vi "cDAQ.vi"(9 "Tipo motore":refnum<vi>, 10 "simulazione?":bool=TRUE, 11 "Dati Targa per calcoli":refnum<vi>) -> (0 "error out":errorcluster)   [LabVIEW 2019]
uses:
  <resource>/objmgr/daqmx.rc
  SET SINGLE DO.ctl
  SET SINGLE AO.ctl
  DO List.ctl
  AO List.ctl
  <vilib>/Analysis/NI_AALBase.lvlib
  <vilib>/Analysis/baseanly.llb/Mean (DBL).vi
  SET ARRAY DO.ctl
  SubVI/Global RPM simulati.vi
  SubVI/Global Coppia letta.vi
  <vilib>/DAQmx/read.llb/DAQmx Read (Counter DBL 1Chan 1Samp).vi
  <vilib>/DAQmx/create/channels.llb/DAQmx Create Channel (CI-Position-Angular Encoder).vi
  <vilib>/DAQmx/configure/timing.llb/DAQmx Timing (Implicit).vi
  <vilib>/DAQmx/create/channels.llb/DAQmx Create Channel (CI-Frequency).vi
  <vilib>/DAQmx/configure/timing.llb/DAQmx Timing (Sample Clock).vi
  <vilib>/DAQmx/create/channels.llb/DAQmx Create Channel (AO-Voltage-Basic).vi
  <vilib>/DAQmx/create/channels.llb/DAQmx Create Channel (AI-Voltage-Basic).vi
  <vilib>/DAQmx/create/channels.llb/DAQmx Create Channel (DO-Digital Output).vi
  <vilib>/DAQmx/create/channels.llb/DAQmx Create Channel (AI-Temperature-Thermocouple).vi
  <vilib>/DAQmx/create/channels.llb/DAQmx Create Channel (DI-Digital Input).vi
  <vilib>/DAQmx/write.llb/DAQmx Write (Analog 1D DBL NChan 1Samp).vi
  <vilib>/DAQmx/read.llb/DAQmx Read (Analog 1D DBL NChan 1Samp).vi
  <vilib>/DAQmx/read.llb/DAQmx Read (Digital 1D Bool 1Chan 1Samp).vi
  <vilib>/DAQmx/read.llb/DAQmx Read (Analog 1D Wfm NChan NSamp).vi
  SubVI/EXIT.vi
  <vilib>/DAQmx/write.llb/DAQmx Write (Digital 1D Bool 1Chan 1Samp).vi
  SubVI/angle global.vi
  SET ARRAY AO.ctl
  controls/statoDO_Cdaq.ctl
panel:
  out "Waveform Chart 2":dbl(graph)
  out "x-y":u32
  out "t ciclo effettivo AO":u32
  out "error out 3":errorcluster
  out "Cnom 2":dbl
  out "Waveform Chart 3":dbl(graph)
  out "error CTR 2":errorcluster
  out "error Angle 2":errorcluster
  out "error out 2":errorcluster
  out "t ciclo effettivo ai":u32
  in  "Time filtro(s)":dbl=0.8 format="%#_13g"
  in  "Tab Control":T1(tab)
  in  "counter 4":tag="C2017003Mod7/ctr1"
  in  "counter 3":tag="C2017003Mod7/ctr3"
  in  "stop":bool
  in  "lines 32DI":tag="C2017003Mod1/port0/line0:31"
  in  "physical channels 4TC":tag="C2017003Mod5/ai0:3, C2017003Mod6/ai0:3"
  in  "lines 32DO":tag="C2017003Mod2/port0/line0:31"
  in  "physical channels 4AO":tag="C2017003Mod4/ao0:3"
  in  "physical channels":tag="C2017003Mod3/ai0:3"
  in  "counter 2":tag="C2017003Mod7/ctr0"
  in  "counter":tag="C2017003Mod7/ctr2"
  in  "SET DO":bool
  in  "Cluster SET AO":T2
  in  "SET AO":bool
  in  "Array DO":T5
  out "statoAO":T8
  out "AI":T9
  out "Termocoppie":T10
  out "angle1":bool
  out "freq":dbl format="%0.2f"
  out "rpm":dbl
  out "t ciclo effettivo LF 1 cntr":u32
  out "statoDO":T11
  out "# pending insert":i32
  out "Numeric":i32
  out "# pending insert 2":i32
  out "angle2":bool
  out "freq 2":dbl format="%0.2f"
  out "rpm 2":dbl
  out "t ciclo effettivo LF 1 cntr 2":u32
  out "error DI":errorcluster
  out "error TC":errorcluster
  out "error DO":errorcluster
  out "error AO":errorcluster
  out "error AI":errorcluster
  out "error Angle":errorcluster
  out "error CTR":errorcluster
  out "XY Graph":cluster{"X":dbl, "Y":dbl}[](graph)
  out "Waveform Chart":waveform(dbl)(graph)
  in  "Boolean":bool
  out "Cnom":dbl
  out "String":string
  in  "EXIT":bool
  in  "STOP GENERALE 2":bool
  # "STATO INGRESSI"
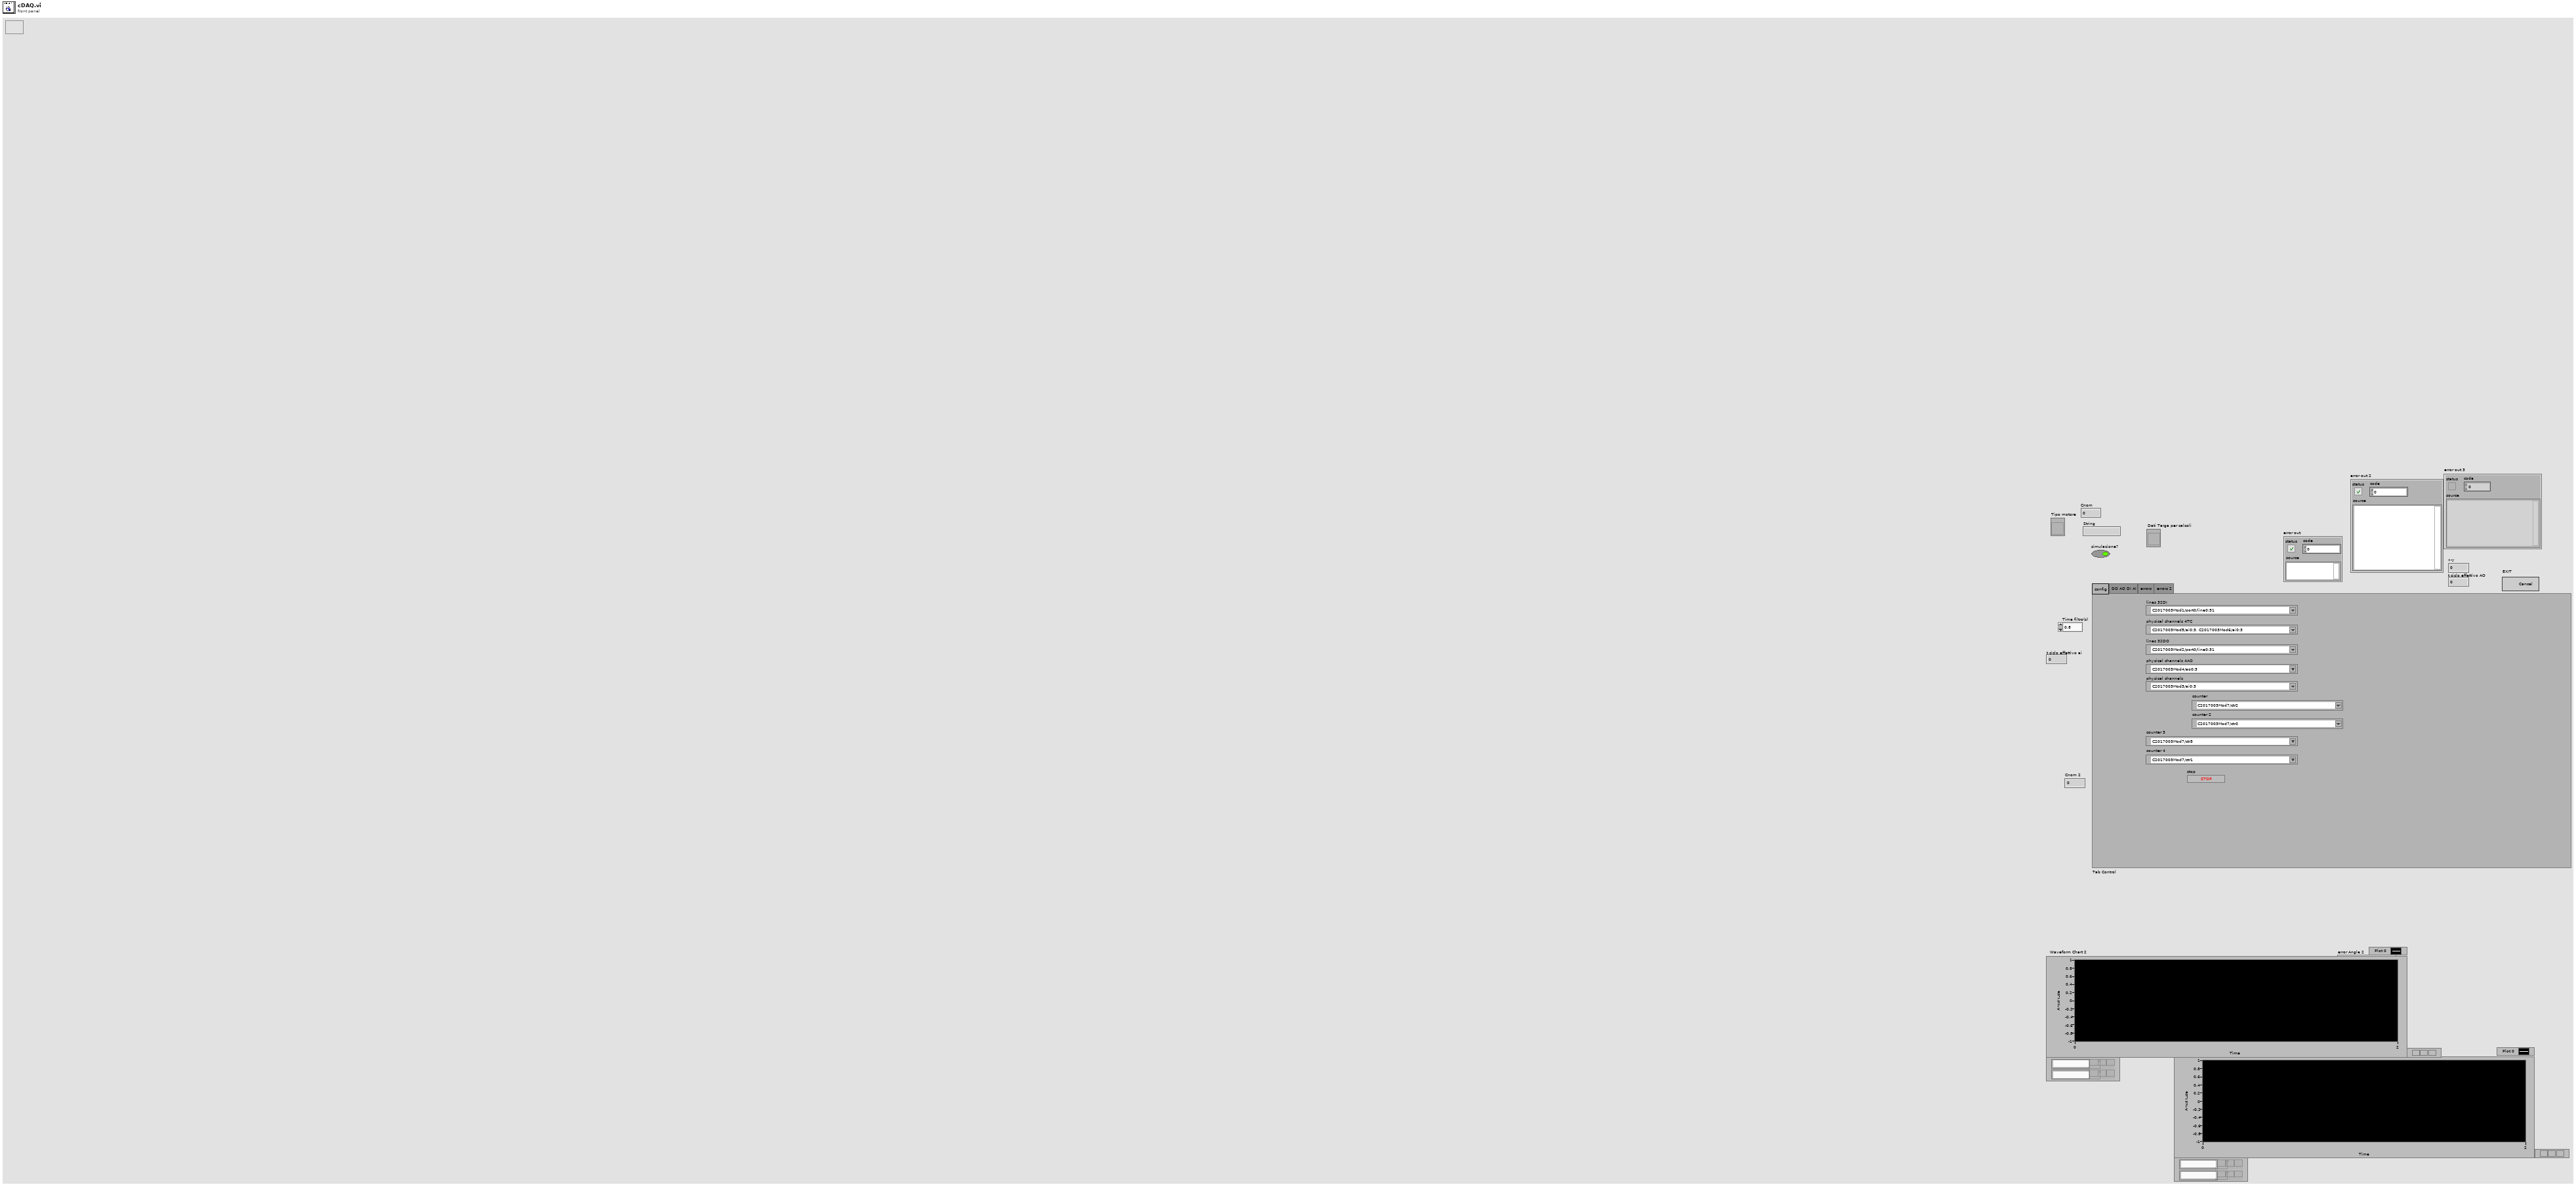
[diagram p1: front panel]
types:
  T1 = enum32{"config", "DO AO DI AI", "errors", "errors 2"}
  T2 = typedef "SET ARRAY AO.ctl" = T3[]
  T3 = typedef "SET SINGLE AO.ctl" = cluster{"AO":T4, "Value":dbl}
  T4 = typedef "AO List.ctl" = enum16{"OFF: ALL AO", "RIF VEL FRENO 1", "RIF VEL FRENO 2", "RIF VEL FRENO 3", "RIF COPPIA FRENO 1", "RIF COPPIA FRENO 2", "RIF COPPIA FRENO 3", "RIF V ALIM 1", "RIF F ALIM 1", "RIF V ALIM 2", "RIF F ALIM 2", "RIF V ALIM 3", "RIF F ALIM 3", "RIF V ALIM 4", "RIF F ALIM 4", "FORZA AO PLC 3", "FORZA AO PLC 2", "FORZA AO PLC 1", "FORZA AO cDAQ", "Configura alimentatore keb", "Tempo rampa keb", "Condensatori", "Exit"}
  T5 = typedef "SET ARRAY DO.ctl" = T6[]
  T6 = typedef "SET SINGLE DO.ctl" = cluster{"DO":T7, "Value":bool}
  T7 = typedef "DO List.ctl" = enum16{"OFF: ALL DO", "*ABILITA freno 1", "*ABILITA freno 2", "*ABILITA freno 3", "*START freno 1", "*START freno 2", "*START freno 3", "*STOP freno 1", "*STOP freno 3", "*STOP freno 2", "*Senso rot freno 1", "*Senso rot freno 2", "*Senso rot freno 3", "*Ctrl velocità freno 1", "*Ctrl velocità freno 2", "*Ctrl velocità freno 3", "*Ctrl coppia freno 1", "*Ctrl coppia freno 2", "*Ctrl coppia freno 3", "*ABILITA alimentatore 1", "*ABILITA alimentatore 2", "*ABILITA alimentatore 3", "*ABILITA alimentatore 4", "*START alimentatore 1", "*START alimentatore 2", "*START alimentatore 3", "*START alimentatore 4", "*STOP alimentatore 1", "*STOP alimentatore 2", "*STOP alimentatore 3", "*STOP alimentatore 4", "SENSO ROT alimentatore 1", "SENSO ROT alimentatore 2", "Abilita LEM 1000A", "Abilita LEM 300A", "Abilita sensori EXT WT", "B1 Seleziona linea 1", "B1 Seleziona linea 2", "B1 Seleziona linea 3", "B1 Seleziona linea 4", "B1 Seleziona linea 5", "B2 Seleziona linea 1", "B2 Seleziona linea 2", "B2 Seleziona linea 3", "B2 Seleziona linea 4", "B2 Seleziona linea 5", "*Reset allarmi", "*Start potenza AC", "*Stop potenza AC", "*Start potenza DC", "*Stop potenza DC", "*Start potenza DC eccit", "*Stop pontenza DC eccit", "Bypass res meter", "2nd canale res meter", "Enable res meter", "*Abilit teler ramo WT", "*Abil teler ramo princ Resit", "*Abil teler ramo 1 Resist", "*Abil teler ramo 2 Resist", "*Abil teler ramo 3 Resist", "*Abil cortocirc avvolgim", "*Controllo torsiometro B1", "*Controllo Torsiom B2", "*Scala torsiometro B1", "*Scala torsiometro B2", "*Collaudo in corso", "*Allarme presente", "Abilitazione elettroserratura", "Exit", "*Abilita collaudo", "*Abilita potenza trifase", "*Abilita potenza monofase", "*Abilita potenza DC", "*Abilita potenza DC eccit", "*Disabilita teleruttori potenza", "Set teleruttori prova a freddo", "Prova a freddo monofase", "Watchdog", "Forza DO PLC 3", "Forza DO PLC 2", "Forza DO PLC 1", "Forza DO cDAQ", "Scala 2000(T) 200(F) res meter", "Seleziona banco 1", "Seleziona banco 2", "Comando azionam in blocco", "Comando azionam reset", "Sensibilità freno 16 32 nm", "Reset Allarmi", "Carico res - Ramo 1", "Carico res - Ramo 2", "Carico res - Ramo 3", "Carico res - Ramo 4", "Carico res - Ramo 5", "Carico res - Ramo 6", "Carico res - Ramo 7", "Carico res - Ramo 8", "Carico res - Ramo 9", "Carico res - Ramo 10", "Carico res - Ramo 11", "Carico res - Start ventilatore", "Carico res - Stop ventilatore", "Abilita potenza solo freno", "Abilita AFE + freno trasc", "Abilita potenza carico resistivo", "Chiudi potenza AFE", "Apri potenza AFE", "Start AFE", "Config Banco2 TDE", "Misura diretto WT", "Ripristina centralina protezioni", "Abilita Scrittura Dati Keb"}
  T8 = cluster{"V eccitaz":dbl, "I eccitaz":dbl, "Rif vel freno":dbl, "Rif coppia freno":dbl}
  T9 = cluster{"Torsiometro":dbl, "V eccitazione":dbl, "I eccitazione":dbl, "Scorta":dbl}
  T10 = cluster{"TC 1":dbl, "TC 2":dbl, "TC 3":dbl, "Tamb (°C)":dbl, "TC 4":dbl, "TC 5":dbl, "TC 6":dbl, "Tamb (°C) 2":dbl}
  T11 = typedef "statoDO_Cdaq.ctl" = cluster{"Scorta 0":bool, "Scorta 1":bool, "Scorta 2":bool, "Scorta 3":bool, "Scorta 4":bool, "Scorta 5":bool, "Scorta 6":bool, "Scorta 7":bool, "Scorta 8":bool, "Scorta 9":bool, "Scorta 10":bool, "Scorta 11":bool, "Scorta 12":bool, "Scorta 13":bool, "Scorta 14":bool, "Scorta 15":bool, "Scorta 16":bool, "Scorta 17":bool, "Scorta 18":bool, "Scorta 19":bool, "Scorta 20":bool, "Scorta 21":bool, "Scorta 22":bool, "Scorta 23":bool, "Scorta 24":bool, "Scorta 25":bool, "Scorta 26":bool, "Scorta 27":bool, "Scorta 28":bool, "Scorta 29":bool, "Scorta 30":bool, "Scorta 31":bool}
  T12 = typedef "Dati targa per calcoli.ctl" = cluster{"trifase":cluster{"I nom (A)":dbl, "C nom (Nm)":dbl, "Npoli":dbl, "V nom (V)":dbl, "RPM nom":dbl}, "Monofase":cluster{"I nom (A)":dbl, "C nom (Nm)":dbl, "Npoli":dbl, "V nom (V)":dbl, "RPM nom":dbl}, "Dc":cluster{"I nom (A)":dbl, "C nom (Nm)":dbl, "V nom (V)":dbl, "RPM nom":dbl}}
  T13 = cluster{"[0]":dbl, "[1]":dbl, "[2]":dbl, "[3]":dbl}
  T14 = cluster{"Motore monofase abil":bool, "Motore trifase abil":bool, "Uscita generale abil":bool, "2nd ch res meter abil":bool, "TA selezionati":bool, "Pulsante Start prova":bool, "Pulsante Stop prova":bool, "Pulsante Reset allarmi":bool, "Secondari TA aperti":bool, "Res meter abil":bool, "Scorta 1":bool, "Scorta 2":bool, "Scorta 3":bool, "Scorta 4":bool, "Scorta 5":bool, "Scorta 6":bool, "Scorta 7":bool, "Scorta 8":bool, "Scorta 9":bool, "Scorta 10":bool, "Scorta 11":bool, "Scorta 12":bool, "Scorta 13":bool, "Scorta 14":bool, "Scorta 15":bool, "Scorta 16":bool, "Scorta 17":bool, "Scorta 18":bool, "Scorta 19":bool, "Scorta 20":bool, "Scorta 21":bool, "Scorta 22":bool}
  T15 = cluster{"data[0]":dbl, "data[1]":dbl, "data[2]":dbl, "data[3]":dbl, "data[4]":dbl, "data[5]":dbl, "data[6]":dbl, "data[7]":dbl}
  T16 = cluster{"[0]":bool, "[1]":bool, "[2]":bool, "[3]":bool, "[4]":bool, "[5]":bool, "[6]":bool, "[7]":bool, "[8]":bool, "[9]":bool, "[10]":bool, "[11]":bool, "[12]":bool, "[13]":bool, "[14]":bool, "[15]":bool, "[16]":bool, "[17]":bool, "[18]":bool, "[19]":bool, "[20]":bool, "[21]":bool, "[22]":bool, "[23]":bool, "[24]":bool, "[25]":bool, "[26]":bool, "[27]":bool, "[28]":bool, "[29]":bool, "[30]":bool, "[31]":bool}
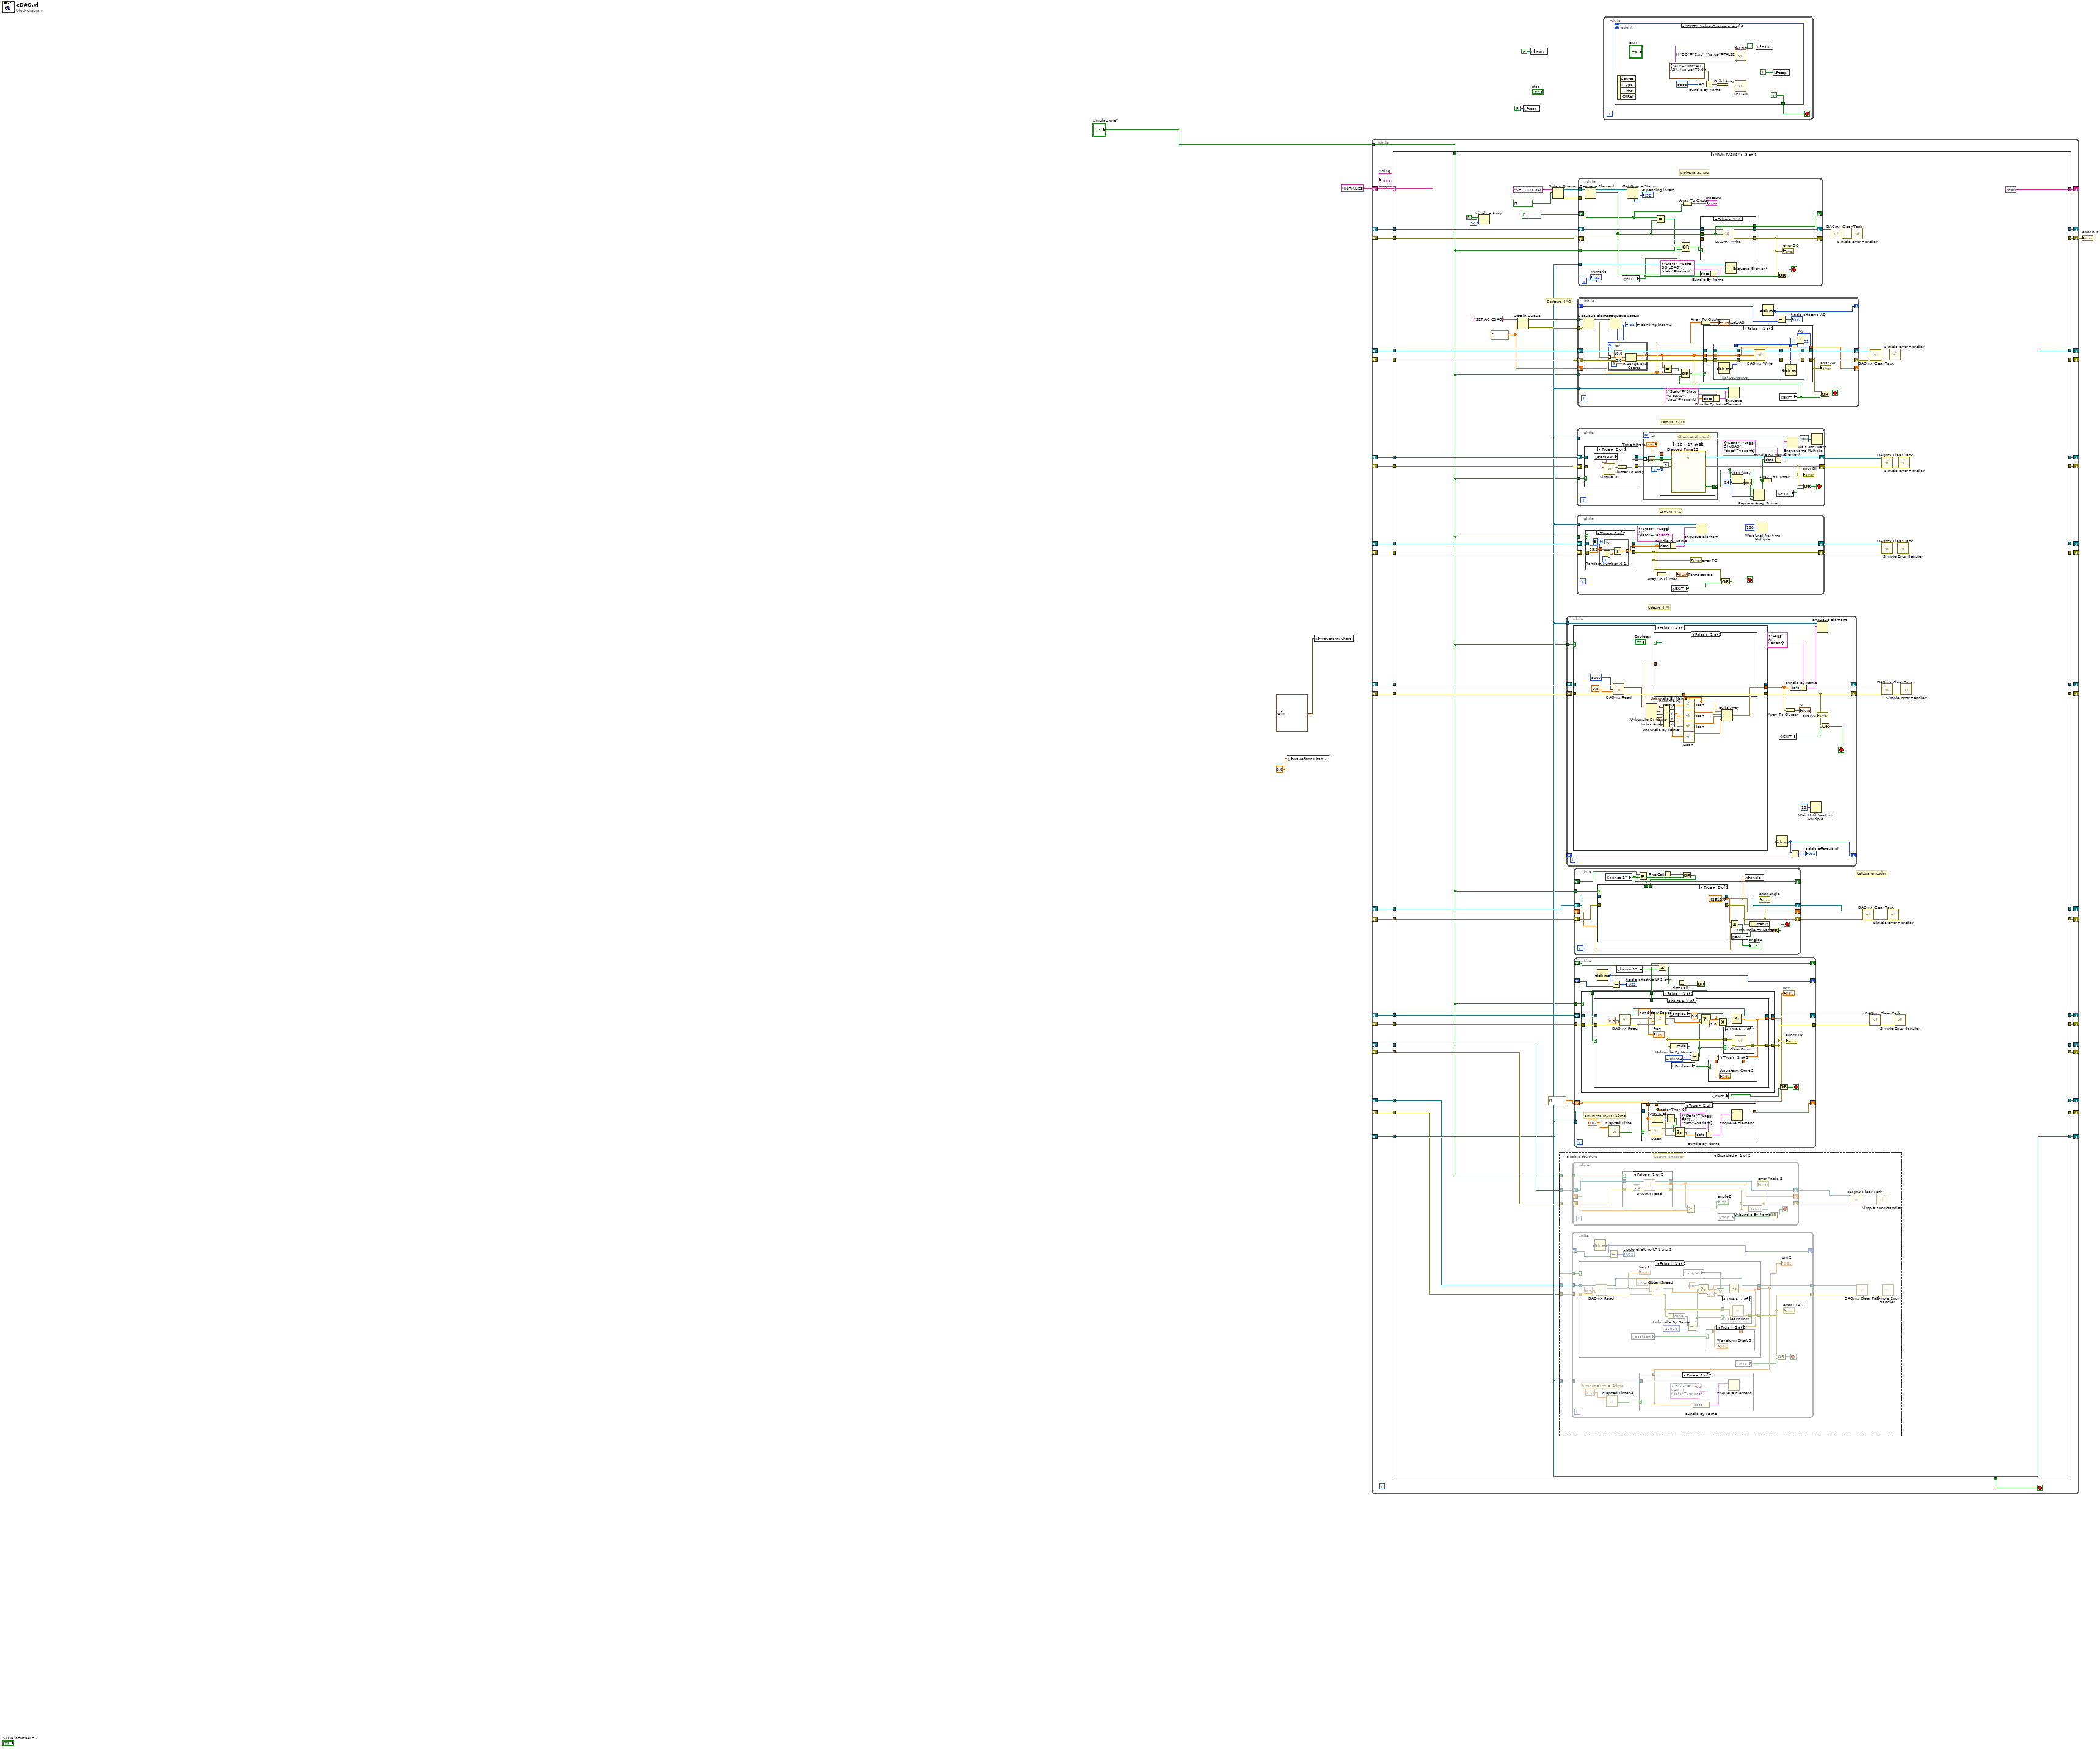
[diagram p0: block diagram]
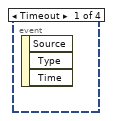
[diagram p2: hidden frame]
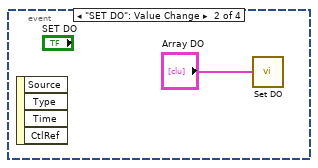
[diagram p3: hidden frame]
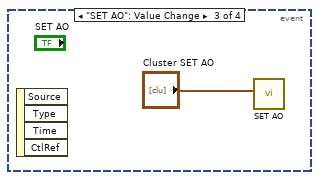
[diagram p4: hidden frame]
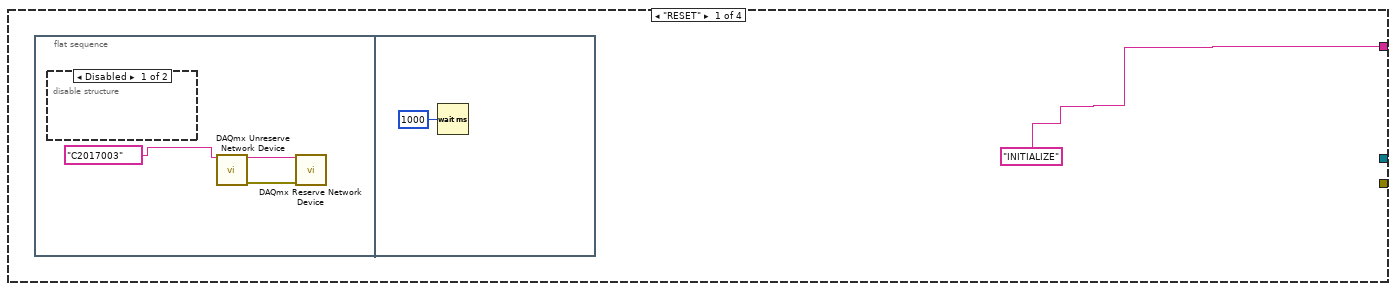
[diagram p5: hidden frame]
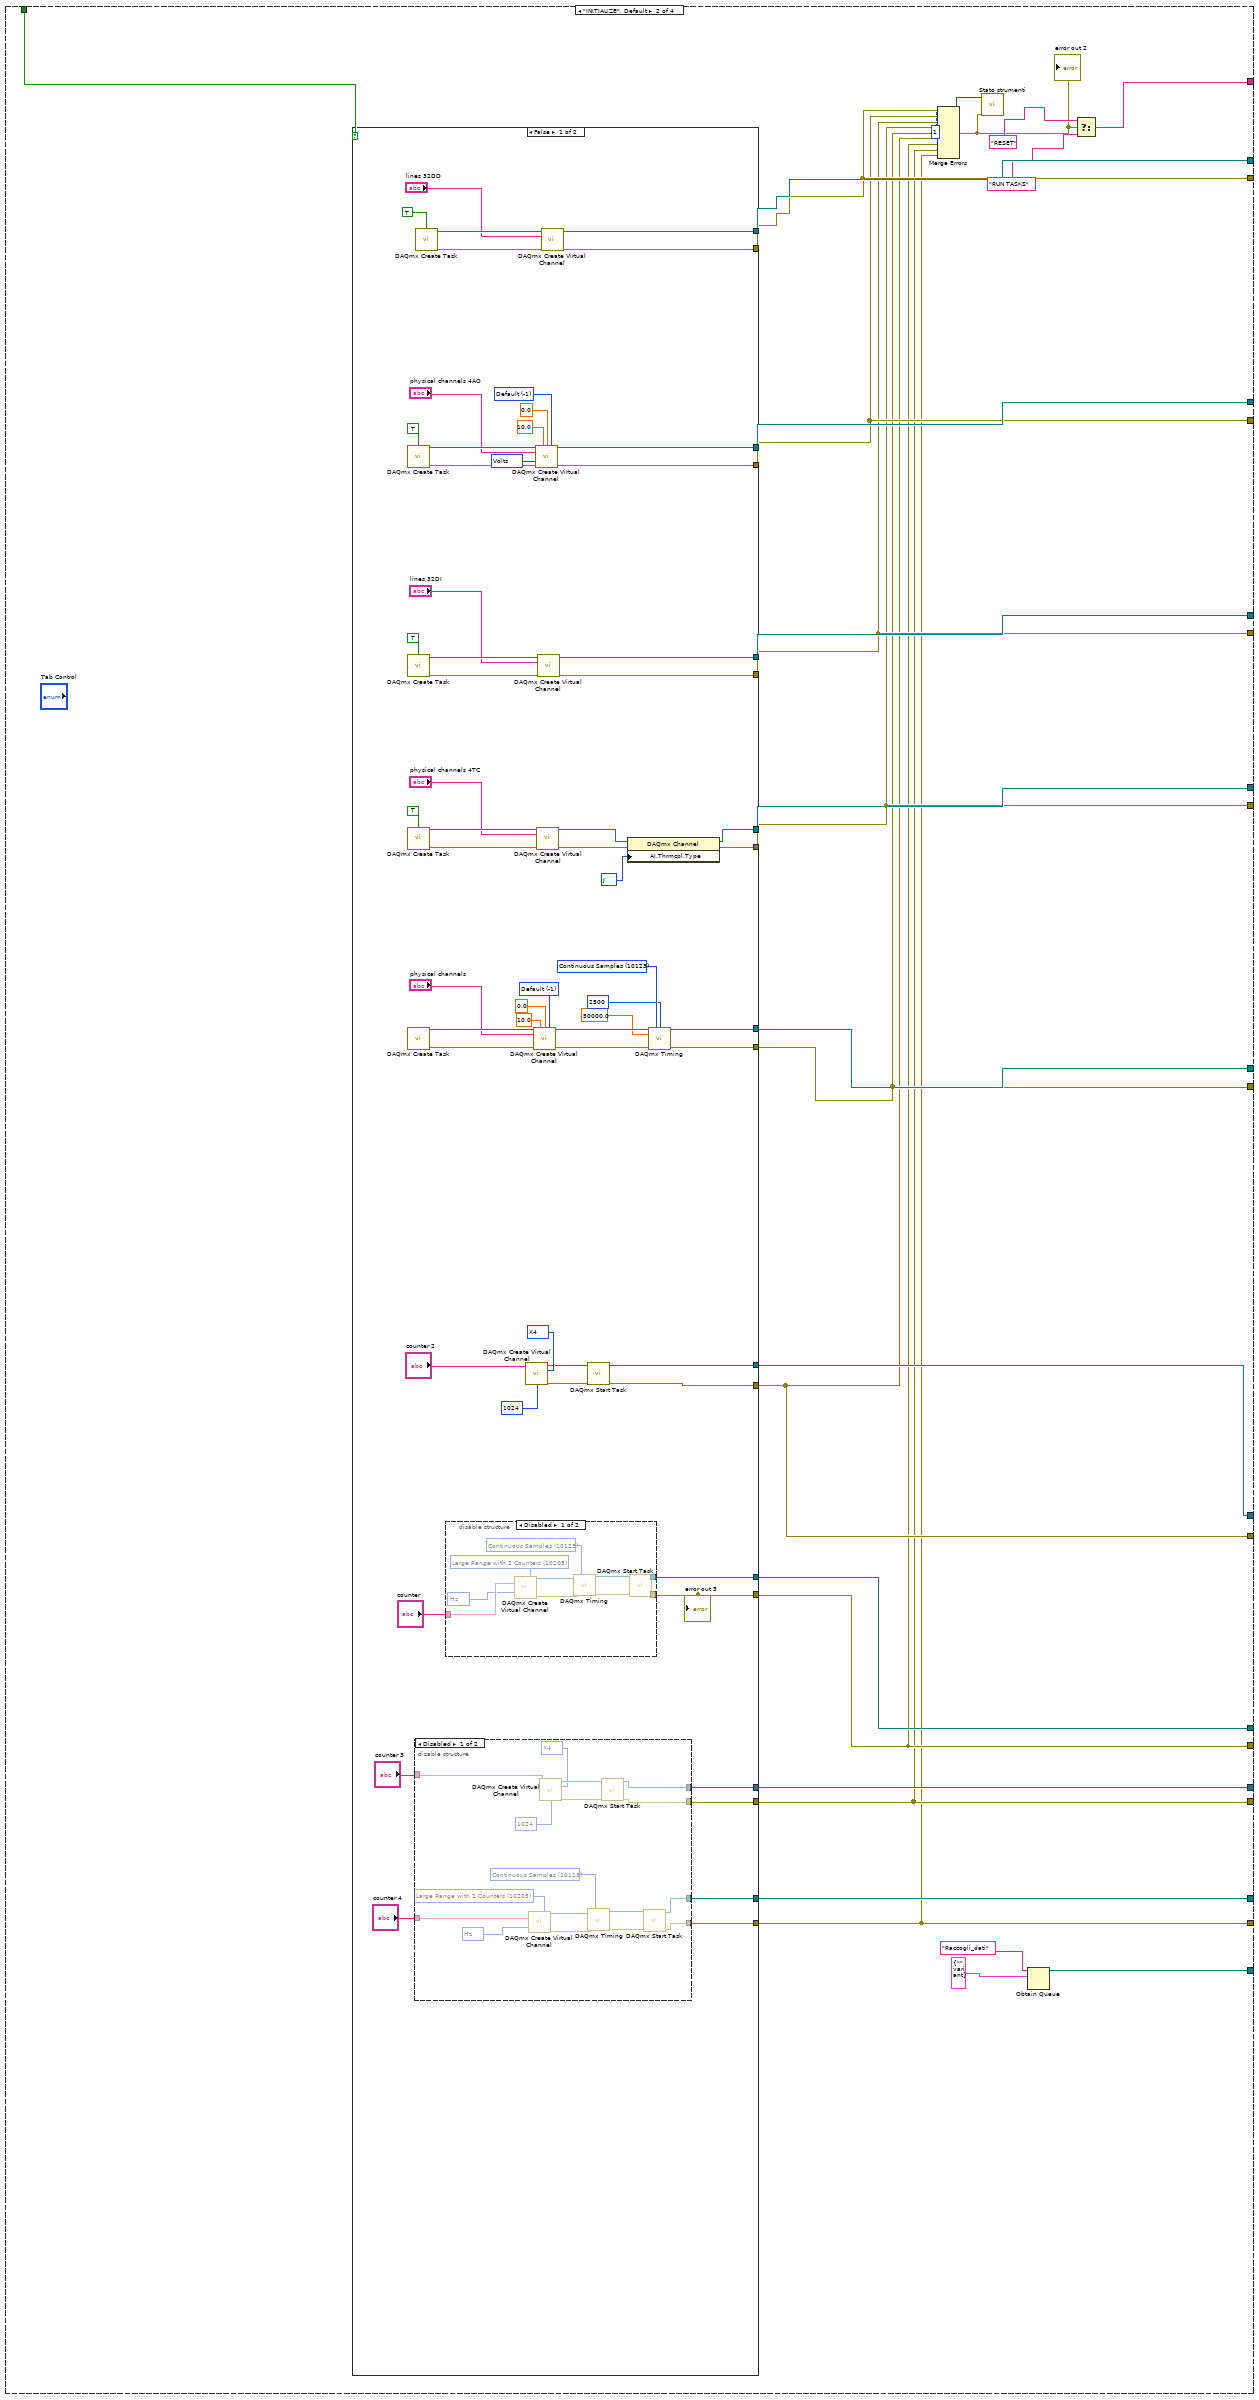
[diagram p7: hidden frame]
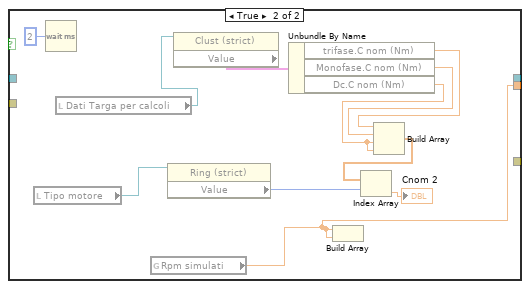
[diagram p13: hidden frame]
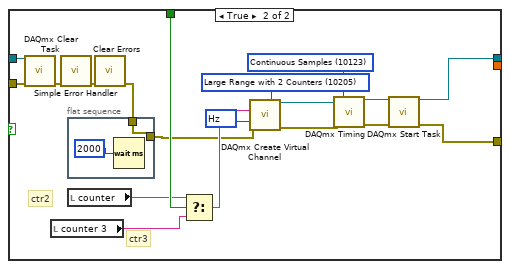
[diagram p19: hidden frame]
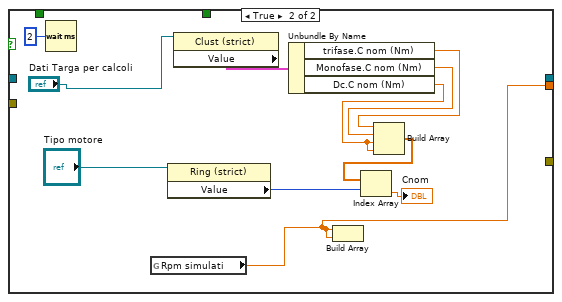
[diagram p20: hidden frame]
diagram:
  n1 = local write "Waveform Chart 2"(0.0 ("Speed [RPM]")) -> ()
  n2 = local write "Waveform Chart"(waveform(dbl) {"t0"=timestamp(0 s since 1904-01-01), "dt"=1.0, "Y"=[]} ("waveform")) -> ()
  n3 = while {
    tunnel: "simulazione?" -> [w42]
    shift-right: [w33] -> _
    shift-left: "INITIALIZE" -> [w34]
    shift-right: [w32] -> _
    shift-left: _ -> [w48]
    shift-right: [w31] -> w3
    shift-left: _ -> [w35]
    shift-right: [w30] -> _
    shift-left: _ -> [w45]
    shift-right: [w29] -> _
    shift-left: _ -> [w36]
    shift-right: [w28] -> _
    shift-left: _ -> [w49]
    shift-right: [w27] -> _
    shift-left: _ -> [w37]
    shift-right: [w26] -> _
    shift-left: _ -> [w47]
    shift-right: [w25] -> _
    shift-left: _ -> [w38]
    shift-right: [w24] -> _
    shift-left: _ -> [w46]
    shift-right: [w23] -> _
    shift-left: _ -> [w39]
    shift-right: [w22] -> _
    shift-left: _ -> [w44]
    shift-right: [w21] -> _
    shift-left: _ -> [w40]
    shift-right: [w20] -> _
    shift-left: _ -> [w43]
    shift-right: [w19] -> _
    shift-left: _ -> [w41]
    shift-right: [w18] -> _
    shift-left: _ -> [w17]
    shift-right: [w15] -> _
    shift-left: _ -> [w11]
    shift-right: [w14] -> _
    shift-left: _ -> [w10]
    shift-right: [w13] -> _
    shift-left: _ -> [w9]
    shift-right: [w12] -> _
    shift-left: _ -> [w8]
    stop <- w16 stop-if-true
    n4 = case shown="\"RUN TASKS\"" w34 {
      tunnel: w49 -> [_ _ w222 _]
      tunnel: w48 -> [_ _ w218 _]
      tunnel: w47 -> [_ _ w216 _]
      tunnel: w46 -> [_ _ w213 _]
      tunnel: w45 -> [_ _ w208 _]
      tunnel: w44 -> [_ _ w202 _]
      tunnel: w43 -> [_ _ w201 _]
      tunnel: w42 -> [_ w74 w172 _]
      tunnel: w41 -> [_ _ w200 _]
      tunnel: w40 -> [_ _ w199 _]
      tunnel: w39 -> [_ _ w198 _]
      tunnel: w38 -> [_ _ w197 _]
      tunnel: w37 -> [_ _ w196 _]
      tunnel: w36 -> [_ _ w195 _]
      tunnel: w35 -> [_ _ w194 _]
      tunnel: ["INITIALIZE" w61 "EXIT" _] -> w33
      tunnel: [_ w81 _ _] -> w32
      tunnel: [_ w70 _ _] -> w31
      tunnel: [_ w80 _ _] -> w30
      tunnel: [_ w69 _ _] -> w29
      tunnel: [_ w79 _ _] -> w28
      tunnel: [_ w68 _ _] -> w27
      tunnel: [_ w78 _ _] -> w26
      tunnel: [_ w67 _ _] -> w25
      tunnel: [_ w77 _ _] -> w24
      tunnel: [_ w66 _ _] -> w23
      tunnel: [_ w76 _ _] -> w22
      tunnel: [_ w65 _ _] -> w21
      tunnel: [_ w75 _ _] -> w20
      tunnel: [_ w64 _ _] -> w19
      tunnel: [_ w71 w173 _] -> w18
      tunnel: w17 -> [_ _ w173 w778]
      tunnel: [_ _ _ TRUE] -> w16
      tunnel: [_ w58 _ _] -> w15
      tunnel: [_ w56 _ _] -> w14
      tunnel: [_ w57 _ _] -> w13
      tunnel: [_ w55 _ _] -> w12
      tunnel: w11 -> [_ _ w175 _]
      tunnel: w10 -> [_ _ w174 _]
      tunnel: w9 -> [_ _ w171 _]
      tunnel: w8 -> [_ _ w170 _]
      frame "RESET" {
        n5 = flat-sequence {
          frame #0 {
            n6 = disable-structure shown="Disabled" {
              frame Disabled {
              }
              frame Enabled {
              }
            }
            n7 = call <vilib>:"DAQmx Unreserve Network Device.vi"("device in"=tag "C2017003") -> ("device out"=w52:tag, "error out"=w51:errorcluster)  [unwired: 13 in]
            n8 = call <vilib>:"DAQmx Reserve Network Device.vi"("device in"=w52, "error in"=w51) -> ()  [unwired: 12 in, 2 out]
          }
          frame #1 {
            n9 = Wait (ms)(milliseconds to wait=u32 1000) -> ()  [unwired: 1 out]
          }
        }
      }
      frame "INITIALIZE", Default {
        n10 = case shown="False" w74 {
          tunnel: [w137 _] -> w79
          tunnel: [w136 _] -> w68
          tunnel: [w128 _] -> w81
          tunnel: [w127 _] -> w70
          tunnel: [w123 _] -> w78
          tunnel: [w121 _] -> w67
          tunnel: [w97 _] -> w66
          tunnel: [w99 _] -> w77
          tunnel: [w114 _] -> w69
          tunnel: [w109 _] -> w80
          tunnel: [w104 _] -> w76
          tunnel: [w103 _] -> w65
          tunnel: [w101 _] -> w75
          tunnel: [w102 _] -> w64
          tunnel: [w85 _] -> w58
          tunnel: [w84 _] -> w56
          tunnel: [w83 _] -> w57
          tunnel: [w82 _] -> w55
          frame False {
            w93 = 10092 items=["X1"=10090, "X2"=10091, "X4"=10092, "Two Pulse Counting"=10313] ("decoding type")
            w95 = 10123 items=["Finite Samples"=10178, "Continuous Samples"=10123, "Hardware Timed Single Point"=12522] ("sample mode")
            w105 = -1 items=["Default"=-1, "RSE"=10083, "Differential"=10106, "Pseudodifferential"=12529] ("output terminal configuration")
            w106 = 10348 items=["Volts"=10348, "From Custom Scale"=10065] ("units")
            w117 = -1 items=["Default"=-1, "RSE"=10083, "NRSE"=10078, "Differential"=10106, "Pseudodifferential"=12529] ("input terminal configuration")
            w125 = 10072 items=["J"=10072, "K"=10073, "N"=10077, "R"=10082, "S"=10085, "T"=10086, "B"=10047, "E"=10055] ("AI.Thrmcpl.Type")
            n11 = call <vilib>:"DAQmx Create Task.vi"("auto cleanup"=TRUE) -> ("task out"=w112:refnum<k21>, "error out"=w113:errorcluster)  [unwired: 13 in]
            n12 = call <vilib>:"DAQmx Create Task.vi"("auto cleanup"=TRUE) -> ("task out"=w140:refnum<k21>, "error out"=w138:errorcluster)  [unwired: 13 in]
            n13 = call <vilib>:"DAQmx Create Task.vi"("auto cleanup"=TRUE) -> ("task out"=w134:refnum<k21>, "error out"=w135:errorcluster)  [unwired: 13 in]
            n14 = call <vilib>:"DAQmx Create Task.vi"() -> ("task out"=w120:refnum<k21>, "error out"=w115:errorcluster)  [unwired: 14 in]
            n15 = disable-structure shown="Disabled" {
              disable-tunnel: "counter 3" -> [w157 _]
              disable-tunnel: "counter 4" -> [w156 _]
              disable-tunnel: [w155 _] -> w85
              disable-tunnel: [w154 _] -> w84
              disable-tunnel: [w153 _] -> w83
              disable-tunnel: [w152 _] -> w82
              frame Disabled {
                w167 = 10373 items=["Hz"=10373, "Ticks"=10304, "From Custom Scale"=10065] ("units")
                w163 = 10092 items=["X1"=10090, "X2"=10091, "X4"=10092, "Two Pulse Counting"=10313] ("decoding type")
                w162 = 10205 items=["Low Frequency with 1 Counter"=10105, "High Frequency with 2 Counters"=10157, "Large Range with 2 Counters"=10205] ("measurement method")
                w158 = 10123 items=["Finite Samples"=10178, "Continuous Samples"=10123, "Hardware Timed Single Point"=12522] ("sample mode")
                n16 = call-poly <vilib>:"DAQmx Create Virtual Channel.vi"("measurement method"=w162, "counter"=w156, "units"=w167) -> ("task out"=w160:refnum<k21>, "error out"=w159:errorcluster)  [unwired: 11 in]
                n17 = call-poly <vilib>:"DAQmx Create Virtual Channel.vi"("counter"=w157, "decoding type"=w163, "pulses per revolution"=u32 1024) -> ("task out"=w165:refnum<k21>, "error out"=w166:errorcluster)  [unwired: 11 in]
                n18 = call-poly <vilib>:"DAQmx Timing.vi"("task/channels in"=w160, "sample mode"=w158, "error in"=w159) -> ("task out"=w168:refnum<k21>, "error out"=w161:errorcluster)  [unwired: 11 in]
                n19 = call <vilib>:"DAQmx Start Task.vi"("task/channels in"=w165, "error in"=w166) -> ("task out"=w155:refnum<k21>, "error out"=w154:errorcluster)  [unwired: 12 in]
                n20 = call <vilib>:"DAQmx Start Task.vi"("task/channels in"=w168, "error in"=w161) -> ("task out"=w153:refnum<k21>, "error out"=w152:errorcluster)  [unwired: 12 in]
              }
              frame Enabled {
              }
            }
            n21 = call <vilib>:"DAQmx Create Task.vi"("auto cleanup"=TRUE) -> ("task out"=w130:refnum<k21>, "error out"=w129:errorcluster)  [unwired: 13 in]
            n22 = disable-structure shown="Disabled" {
              disable-tunnel: [w151 _] -> w102
              disable-tunnel: [w150 _] -> w101
              disable-tunnel: "counter" -> [w144 _]
              frame Disabled {
                w143 = 10373 items=["Hz"=10373, "Ticks"=10304, "From Custom Scale"=10065] ("units")
                w145 = 10205 items=["Low Frequency with 1 Counter"=10105, "High Frequency with 2 Counters"=10157, "Large Range with 2 Counters"=10205] ("measurement method")
                w149 = 10123 items=["Finite Samples"=10178, "Continuous Samples"=10123, "Hardware Timed Single Point"=12522] ("sample mode")
                n23 = call-poly <vilib>:"DAQmx Create Virtual Channel.vi"("measurement method"=w145, "counter"=w144, "units"=w143) -> ("task out"=w147:refnum<k21>, "error out"=w148:errorcluster)  [unwired: 11 in]
                n24 = call-poly <vilib>:"DAQmx Timing.vi"("task/channels in"=w147, "sample mode"=w149, "error in"=w148) -> ("task out"=w142:refnum<k21>, "error out"=w146:errorcluster)  [unwired: 11 in]
                n25 = call <vilib>:"DAQmx Start Task.vi"("task/channels in"=w142, "error in"=w146) -> ("task out"=w150:refnum<k21>, "error out"=w151:errorcluster)  [unwired: 12 in]
              }
              frame Enabled {
              }
            }
            "error out 3" <- w102
            n26 = call-poly <vilib>:"DAQmx Create Virtual Channel.vi"("counter"="counter 2", "decoding type"=w93, "pulses per revolution"=u32 1024) -> ("task out"=w91:refnum<k21>, "error out"=w90:errorcluster)  [unwired: 11 in]
            n27 = call-poly <vilib>:"DAQmx Create Virtual Channel.vi"("task in"=w120, "maximum value"=10.0, "minimum value"=0.0, "input terminal configuration"=w117, "physical channels"="physical channels", "error in"=w115) -> ("task out"=w100:refnum<k21>, "error out"=w98:errorcluster)  [unwired: 8 in]
            n28 = call-poly <vilib>:"DAQmx Create Virtual Channel.vi"("task in"=w112, "maximum value"=10.0, "minimum value"=0.0, "output terminal configuration"=w105, "physical channels"="physical channels 4AO", "units"=w106, "error in"=w113) -> ("task out"=w109:refnum<k21>, "error out"=w114:errorcluster)  [unwired: 7 in]
            n29 = call-poly <vilib>:"DAQmx Create Virtual Channel.vi"("task in"=w134, "physical channels"="physical channels 4TC", "error in"=w135) -> ("task out"=w124:refnum<k21>, "error out"=w122:errorcluster)  [unwired: 11 in]
            n30 = call-poly <vilib>:"DAQmx Create Virtual Channel.vi"("task in"=w140, "lines"="lines 32DI", "error in"=w138) -> ("task out"=w137:refnum<k21>, "error out"=w136:errorcluster)  [unwired: 11 in]
            n31 = call-poly <vilib>:"DAQmx Create Virtual Channel.vi"("task in"=w130, "lines"="lines 32DO", "error in"=w129) -> ("task out"=w128:refnum<k21>, "error out"=w127:errorcluster)  [unwired: 11 in]
            n32 = call <vilib>:"DAQmx Start Task.vi"("task/channels in"=w91, "error in"=w90) -> ("task out"=w104:refnum<k21>, "error out"=w103:errorcluster)  [unwired: 12 in]
            n33 = property class="DAQmx Channel"(reference=w124, error in=w122, "AI.Thrmcpl.Type"=w125) -> (reference out=w123:refnum<k21>, error out=w121:errorcluster)
            n34 = call-poly <vilib>:"DAQmx Timing.vi"("task/channels in"=w100, "sample mode"=w95, "samples per channel"=2500, "rate"=50000.0, "error in"=w98) -> ("task out"=w99:refnum<k21>, "error out"=w97:errorcluster)  [unwired: 9 in]
          }
          frame True {
          }
        }
        n35 = Merge Errors(w70, w69, w68, w67, w66, w65, w64, w56, w55) -> (w60:errorcluster)
        "error out 2" <- w60
        n36 = call "Stato strumenti.vi"("error in (no error)"=w60, "Indice"=1) -> ()  [unwired: 10 in]
        n37 = Obtain Queue(name (unnamed)="Raccogli_dati", element data type=cluster{"Stato":string, "dato":variant} {"Stato"="", "dato"=variant} ("Cluster")) -> (queue out=w71:refnum<queue>)  [unwired: 3 in, 2 out]
        n38 = Select(t="RESET", s=w60, f="RUN TASKS") -> (s? t:f=w61:string)
      }
      frame "RUN TASKS" {
        w182 = dbl[] []
        # "Scrittura 4AO"
        # "Lettura encoder"
        # "Lettura 4 AI"
        # "Scrittura 32 DO"
        # "Lettura 4TC"
        # "Lettura 32 DI"
        n39 = Initialize Array(FALSE ("Value"), 32 ("dimension size")) -> ()  [unwired: 1 out]
        n40 = Obtain Queue(name (unnamed)="SET AO CDAQ", element data type=w182) -> (queue out=w205:refnum<queue>, error out=w206:errorcluster)  [unwired: 3 in, 1 out]
        n41 = Obtain Queue(name (unnamed)="SET DO CDAQ", element data type=bool[] []) -> (queue out=w210:refnum<queue>, error out=w211:errorcluster)  [unwired: 3 in, 1 out]
        n42 = disable-structure shown="Disabled" {
          disable-tunnel: w175 -> [w231 _]
          disable-tunnel: w174 -> [w230 _]
          disable-tunnel: w173 -> [w226 _]
          disable-tunnel: w172 -> [w225 _]
          disable-tunnel: w171 -> [w224 _]
          disable-tunnel: w170 -> [w223 _]
          frame Disabled {
            # "Lettura encoder"
            n43 = while {
              tunnel: w224 -> [w248]
              tunnel: w223 -> [w247]
              tunnel: [w246] -> w228
              tunnel: [w238] -> w227
              shift-right: [w244] -> _
              shift-left: _ -> [w243]
              tunnel: w226 -> [w242]
              tunnel: w225 -> [w239]
              stop <- w237 stop-if-true
              # "t minimo invio: 10ms"
              n44 = case shown="False" w239 {
                tunnel: w248 -> [w268 _]
                tunnel: w247 -> [w267 _]
                tunnel: [w259 _] -> w246
                tunnel: [w249 w275] -> w235
                tunnel: [w260 _] -> w238
                frame False {
                  n45 = call-poly <vilib>:"DAQmx Read.vi"("task/channels in"=w268, "timeout"=0.5, "error in"=w267) -> ("task out"=w259:refnum<k21>, "data"=w250:dbl, "error out"=w251:errorcluster)  [unwired: 10 in]
                  "freq 2" <- w250
                  n46 = local read "Boolean"() -> (w253:bool)
                  n47 = call "ObtainSpeed.vi"("error in (no error)"=w251, "Pulses per Revolution"=1024.0, "Counter Frequency"=w250) -> ("error out"=w261:errorcluster, "Speed [RPM]"=w256:dbl)  [unwired: 6 in, 1 out]
                  n48 = Unbundle By Name(w261) -> ("code"=w263:i32)
                  n49 = local read "angle1"() -> (w264:bool)
                  n50 = Equal?(x=w263, y=-200284) -> (x = y?=w254:bool)
                  n51 = Select(t=0.0, s=w254, f=w256) -> (s? t:f=w255:dbl)
                  n52 = Multiply(x=w255, y=-1.0) -> (x*y=w258:dbl)
                  n53 = case shown="True" w254 {
                    tunnel: w261 -> [w270 w272]
                    tunnel: [w270 w271] -> w260
                    frame False {
                    }
                    frame True {
                      n54 = call <vilib>:"Clear Errors.vi"("error in (no error)"=w272) -> ("error out"=w271:errorcluster)  [unwired: 5 in, 1 out]
                    }
                  }
                  n55 = Select(t=w255, s=w264, f=w258) -> (s? t:f=w249:dbl)
                  n56 = case shown="True" w253 {
                    tunnel: w249 -> [_ _]
                    tunnel: w249 -> [_ w269]
                    frame False {
                    }
                    frame True {
                      "Waveform Chart 3" <- w269
                    }
                  }
                }
                frame True {
                  n57 = local read "Tipo motore"() -> (w273:refnum<vi>)
                  n58 = Wait (ms)(milliseconds to wait=u32 2) -> ()  [unwired: 1 out]
                  n59 = local read "Dati Targa per calcoli"() -> (w274:refnum<vi>)
                  n60 = global read "Global RPM simulati.vi" "Rpm simulati"() -> (w275:dbl)
                  n61 = property class="Ring (strict)"(reference=w273) -> ("Value"=w278:u16)  [unwired: 1 in, 2 out]
                  n62 = property class="Clust (strict)"(reference=w274) -> ("Value"=w282:T12)  [unwired: 1 in, 2 out]
                  n63 = Unbundle By Name(w282) -> ("trifase.C nom (Nm)"=w281:dbl, "Monofase.C nom (Nm)"=w280:dbl, "Dc.C nom (Nm)"=w276:dbl)
                  n64 = Build Array(w275, w275) -> ()  [unwired: 1 out]
                  n65 = Build Array(w281, w280, w276, w276) -> (w279:dbl[])
                  n66 = Index Array(array=w279, index=w278) -> (element=→"Cnom 2":dbl)
                }
              }
              "rpm 2" <- w235
              "error CTR 2" <- w238
              n67 = Tick Count (ms)() -> (millisecond timer value=w244:u32)
              n68 = call "Elapsed Time34"("Time Target (s)"=0.01) -> ("Time has Elapsed"=w240:bool)  [unwired: 11 in, 7 out]
              n69 = Subtract(x=w244, y=w243) -> (x-y=→"t ciclo effettivo LF 1 cntr 2":u32)
              n70 = case shown="True" w240 {
                tunnel: w242 -> [_ w285]
                tunnel: w235 -> [_ w284]
                frame False {
                }
                frame True {
                  n71 = Bundle By Name(cluster=cluster{"Stato":string, "dato":variant} {"Stato"="Leggi RPM 2", "dato"=variant} ("Cluster"), "dato"=w284) -> (w287:cluster{"Stato":string, "dato":variant})
                  n72 = Enqueue Element(queue=w285, element=w287) -> ()  [unwired: 2 in, 3 out]
                }
              }
              n73 = local read "stop"() -> (w236:bool)
              n74 = Or(x=w238, y=w236) -> (x .or. y?=w237:bool)
            }
            n75 = while {
              shift-right: [w296] -> w234
              shift-left: w231 -> [w298]
              shift-right: [w293] -> w233
              shift-left: w230 -> [w297]
              shift-right: [w295] -> _
              shift-left: _ -> [w294]
              tunnel: w225 -> [w292]
              stop <- w289 stop-if-true
              n76 = case shown="False" w292 {
                tunnel: w298 -> [w304 _]
                tunnel: w297 -> [w303 _]
                tunnel: [w302 _] -> w296
                tunnel: [w300 _] -> w295
                tunnel: [w299 _] -> w293
                frame False {
                  n77 = call-poly <vilib>:"DAQmx Read.vi"("task/channels in"=w304, "timeout"=-1.0, "error in"=w303) -> ("task out"=w302:refnum<k21>, "data"=w300:dbl, "error out"=w299:errorcluster)  [unwired: 10 in]
                }
                frame True {
                }
              }
              "error Angle 2" <- w293
              n78 = Greater Or Equal?(x=w295, y=w294) -> (x >= y?=→"angle2":bool)
              n79 = local read "stop"() -> (w290:bool)
              n80 = Unbundle By Name(w293) -> ("status"=w291:bool)
              n81 = Or(x=w291, y=w290) -> (x .or. y?=w289:bool)
            }
            n82 = call <vilib>:"DAQmx Clear Task.vi"("task in"=w234, "error in"=w233) -> ("error out"=w232:errorcluster)  [unwired: 13 in]
            n83 = call <vilib>:"DAQmx Clear Task.vi"("task in"=w228, "error in"=w227) -> ("error out"=w229:errorcluster)  [unwired: 13 in]
            n84 = call <vilib>:"Simple Error Handler.vi"("error in (no error)"=w232) -> ()  [unwired: 4 in, 5 out]
            n85 = call <vilib>:"Simple Error Handler.vi"("error in (no error)"=w229) -> ()  [unwired: 4 in, 5 out]
          }
          frame Enabled {
          }
        }
        n86 = while {
          shift-right: [w458] -> w214
          shift-left: w213 -> [w460]
          shift-right: [w450] -> w215
          shift-left: w198 -> [w459]
          tunnel: w173 -> [w455]
          tunnel: w172 -> [w452]
          shift-right: [w448] -> _
          shift-left: _ -> [w447]
          stop <- w451 stop-if-true
          n87 = case shown="False" w452 {
            tunnel: w460 -> [w481 _]
            tunnel: w459 -> [w480 _]
            tunnel: [w479 _] -> w450
            tunnel: [w464 _] -> w458
            tunnel: [w477 w507] -> w454
            frame False {
              n88 = call-poly <vilib>:"DAQmx Read.vi"("task/channels in"=w481, "number of samples per channel"=5000, "timeout"=0.5, "error in"=w480) -> ("task out"=w464:refnum<k21>, "data"=w476:waveform(dbl)[], "error out"=w479:errorcluster)  [unwired: 9 in]
              n89 = Index Array(array=w476) -> (element #1=w461:waveform(dbl), element #2=w475:waveform(dbl), element #3=w474:waveform(dbl), element #4=w473:waveform(dbl))  [unwired: 4 in]
              n90 = Unbundle By Name(w461) -> ("Y"=w472:dbl[])
              n91 = Unbundle By Name(w475) -> ("Y"=w471:dbl[])
              n92 = Unbundle By Name(w474) -> ("Y"=w470:dbl[])
              n93 = Unbundle By Name(w473) -> ("Y"=w469:dbl[])
              n94 = call-poly <vilib>:"Mean.vi"("X"=w472) -> ("mean"=w462:dbl)  [unwired: 1 out]
              n95 = case shown="False" "Boolean" {
                tunnel: w461 -> [_ w483]
                tunnel: w462 -> [_ w482]
                frame False {
                }
                frame True {
                  n96 = while {
                    tunnel: w482 -> [w489]
                    shift-right: [w484] -> _
                    shift-left: _ -> [w486]
                    stop <- TRUE stop-if-true
                    n97 = local read "rpm"() -> (w490:dbl)
                    n98 = Absolute Value(x=w490) -> (abs(x)=w488:dbl)
                    n99 = Bundle(w488, "mean"=w489) -> (w485:cluster{dbl, "mean":dbl})  [unwired: 1 in]
                    n100 = Build Array (concatenate)(w486, w485) -> (w484:cluster{dbl, "mean":dbl}[])
                    "XY Graph" <- w484
                  }
                  "Waveform Chart" <- w483
                }
              }
              n101 = call-poly <vilib>:"Mean.vi"("X"=w471) -> ("mean"=w468:dbl)  [unwired: 1 out]
              n102 = call-poly <vilib>:"Mean.vi"("X"=w470) -> ("mean"=w467:dbl)  [unwired: 1 out]
              n103 = call-poly <vilib>:"Mean.vi"("X"=w469) -> ("mean"=w466:dbl)  [unwired: 1 out]
              n104 = Build Array(w462, w468, w467, w466) -> (w477:dbl[])
            }
            frame True {
              w506 = 0.0 ("element")
              n105 = Wait (ms)(milliseconds to wait=u32 50) -> ()  [unwired: 1 out]
              n106 = property on="Scorta 7" class="Bool (strict)"() -> ("Value"=w498:bool)  [unwired: 2 in, 2 out]
              n107 = property on="Scorta 9" class="Bool (strict)"() -> ("Value"=w492:bool)  [unwired: 2 in, 2 out]
              n108 = global read "Global Coppia letta.vi" "C [NM] simulata"() -> (w501:dbl)
              n109 = Select(t=20.0, s=w492, f=200.0) -> (s? t:f=w491:dbl)
              n110 = Select(t=2.0, s=w498, f=20.0) -> (s? t:f=w495:dbl)
              n111 = Divide(x=w501, y=w495) -> (x/y=w502:dbl)
              n112 = Divide(x=w501, y=w491) -> (x/y=w505:dbl)
              n113 = Multiply(x=w502, y=10.0) -> (x*y=w500:dbl)
              n114 = Multiply(x=w505, y=10.0) -> (x*y=w499:dbl)
              n115 = Build Array(w500, w499, w506, w506) -> (w507:dbl[])
            }
          }
          "error AI" <- w450
          n116 = Tick Count (ms)() -> (millisecond timer value=w448:u32)
          n117 = global read "EXIT.vi" "EXIT"() -> (w445:bool)
          n118 = Array To Cluster(array=w454) -> (cluster=→"AI":T13)
          n119 = Subtract(x=w448, y=w447) -> (x-y=→"t ciclo effettivo ai":u32)
          n120 = Bundle By Name(cluster=cluster{"Stato":string, "dato":variant} {"Stato"="Leggi AI", "dato"=variant} ("Cluster"), "dato"=w454) -> (w457:cluster{"Stato":string, "dato":variant})
          n121 = Wait Until Next ms Multiple(millisecond multiple=u32 10) -> ()  [unwired: 1 out]
          n122 = Enqueue Element(queue=w455, element=w457) -> ()  [unwired: 2 in, 3 out]
          n123 = Or(x=w450, y=w445) -> (x .or. y?=w451:bool)
        }
        n124 = while {
          shift-right: [w414] -> w179
          shift-left: w202 -> [w416]
          shift-right: [w413] -> w180
          shift-left: w199 -> [w415]
          shift-right: [w401] -> _
          shift-left: _ -> [w408]
          tunnel: w172 -> [w412]
          shift-right: [w406] -> _
          shift-left: _ -> [w407]
          stop <- w410 stop-if-true
          n125 = global read "Global_scelta_banco" "banco 1?"() -> (w406:bool)
          n126 = Not Equal?(x=w407, y=w406) -> (x != y?=w403:bool)
          n127 = First Call?() -> (First Call?: T/F=w404:bool)
          n128 = Or(x=w404, y=w403) -> (x .or. y?=w402:bool)
          n129 = case shown="True" w412 {
            tunnel: w416 -> [w423 _]
            tunnel: w415 -> [w422 _]
            tunnel: [w421 _] -> w414
            tunnel: [w420 42510.0 ("data")] -> w401
            tunnel: [w419 _] -> w413
            tunnel: w402 -> [w418 _]
            tunnel: w406 -> [w417 _]
            frame False {
              n130 = case shown="True" w418 {
                tunnel: w423 -> [w429 w441]
                tunnel: w422 -> [w428 w442]
                tunnel: [w427 w435] -> w421
                tunnel: [w425 _] -> w420
                tunnel: [w424 w434] -> w419
                tunnel: w417 -> [_ w433]
                frame False {
                  n131 = call-poly <vilib>:"DAQmx Read.vi"("task/channels in"=w429, "timeout"=-1.0, "error in"=w428) -> ("task out"=w427:refnum<k21>, "data"=w425:dbl, "error out"=w424:errorcluster)  [unwired: 10 in]
                }
                frame True {
                  w437 = 10092 items=["X1"=10090, "X2"=10091, "X4"=10092, "Two Pulse Counting"=10313] ("decoding type")
                  # "ctr1"
                  # "ctr0"
                  n132 = local read "counter 2"() -> (w432:tag)
                  n133 = call <vilib>:"DAQmx Clear Task.vi"("task in"=w441, "error in"=w442) -> ("error out"=w443:errorcluster)  [unwired: 13 in]
                  n134 = local read "counter 4"() -> (w430:tag)
                  n135 = call <vilib>:"Simple Error Handler.vi"("error in (no error)"=w443) -> ("error out"=w436:errorcluster)  [unwired: 4 in, 4 out]
                  n136 = Select(t=w432, s=w433, f=w430) -> (s? t:f=w431:tag)
                  n137 = call-poly <vilib>:"DAQmx Create Virtual Channel.vi"("counter"=w431, "decoding type"=w437, "error in"=w436, "pulses per revolution"=u32 1024) -> ("task out"=w439:refnum<k21>, "error out"=w440:errorcluster)  [unwired: 10 in]
                  n138 = call <vilib>:"DAQmx Start Task.vi"("task/channels in"=w439, "error in"=w440) -> ("task out"=w435:refnum<k21>, "error out"=w434:errorcluster)  [unwired: 12 in]
                }
              }
            }
            frame True {
            }
          }
          "error Angle" <- w413
          n139 = Greater Or Equal?(x=w401, y=w408) -> (x >= y?=→"angle1":bool)
          n140 = global read "EXIT.vi" "EXIT"() -> (w405:bool)
          n141 = global write "angle global.vi" "angle"(w401) -> ()
          n142 = Unbundle By Name(w413) -> ("status"=w411:bool)
          n143 = Or(x=w411, y=w405) -> (x .or. y?=w410:bool)
        }
        n144 = while {
          tunnel: w200 -> [w324]
          tunnel: [w315] -> w178
          shift-right: [w321] -> _
          shift-left: _ -> [w320]
          tunnel: w173 -> [w319]
          tunnel: w172 -> [w316]
          shift-right: [w312] -> _
          shift-left: _ -> [w313]
          shift-right: [w323] -> w177
          shift-left: w201 -> [w325]
          shift-right: [w306] -> _
          shift-left: dbl[] [] -> [w307]
          stop <- w314 stop-if-true
          # "t minimo invio: 10ms"
          n145 = Tick Count (ms)() -> (millisecond timer value=w321:u32)
          n146 = call "Elapsed Time"("Time Target (s)"=0.02) -> ("Time has Elapsed"=w317:bool)  [unwired: 11 in, 7 out]
          n147 = Subtract(x=w321, y=w320) -> (x-y=→"t ciclo effettivo LF 1 cntr":u32)
          n148 = global read "Global_scelta_banco" "banco 1?"() -> (w312:bool)
          n149 = Not Equal?(x=w313, y=w312) -> (x != y?=w310:bool)
          n150 = First Call?() -> (First Call?: T/F=w311:bool)
          n151 = Or(x=w311, y=w310) -> (x .or. y?=w309:bool)
          n152 = case shown="False" w316 {
            tunnel: w325 -> [w332 _]
            tunnel: w324 -> [w331 _]
            tunnel: [w329 _] -> w323
            tunnel: [w328 w378] -> w308
            tunnel: [w330 _] -> w315
            tunnel: w309 -> [w327 _]
            tunnel: w312 -> [w326 _]
            frame False {
              n153 = case shown="False" w327 {
                tunnel: w332 -> [w352 w360]
                tunnel: w331 -> [w351 w361]
                tunnel: [w344 w366] -> w330
                tunnel: [w343 w367] -> w329
                tunnel: [w333 _] -> w328
                tunnel: w326 -> [_ w365]
                frame False {
                  n154 = call-poly <vilib>:"DAQmx Read.vi"("task/channels in"=w352, "timeout"=0.5, "error in"=w351) -> ("task out"=w343:refnum<k21>, "data"=w334:dbl, "error out"=w335:errorcluster)  [unwired: 10 in]
                  "freq" <- w334
                  n155 = call "ObtainSpeed.vi"("error in (no error)"=w335, "Pulses per Revolution"=1024.0, "Counter Frequency"=w334) -> ("error out"=w345:errorcluster, "Speed [RPM]"=w340:dbl)  [unwired: 6 in, 1 out]
                  n156 = local read "angle1"() -> (w348:bool)
                  n157 = Unbundle By Name(w345) -> ("code"=w347:i32)
                  n158 = local read "Boolean"() -> (w337:bool)
                  n159 = Equal?(x=w347, y=-200284) -> (x = y?=w338:bool)
                  n160 = Select(t=0.0, s=w338, f=w340) -> (s? t:f=w339:dbl)
                  n161 = Multiply(x=w339, y=-1.0) -> (x*y=w342:dbl)
                  n162 = case shown="True" w338 {
                    tunnel: w345 -> [w354 w356]
                    tunnel: [w354 w355] -> w344
                    frame False {
                    }
                    frame True {
                      n163 = call <vilib>:"Clear Errors.vi"("error in (no error)"=w356) -> ("error out"=w355:errorcluster)  [unwired: 5 in, 1 out]
                    }
                  }
                  n164 = Select(t=w339, s=w348, f=w342) -> (s? t:f=w333:dbl)
                  n165 = case shown="True" w337 {
                    tunnel: w333 -> [_ _]
                    tunnel: w333 -> [_ w353]
                    frame False {
                    }
                    frame True {
                      "Waveform Chart 2" <- w353
                    }
                  }
                }
                frame True {
                  w369 = 10373 items=["Hz"=10373, "Ticks"=10304, "From Custom Scale"=10065] ("units")
                  w370 = 10205 items=["Low Frequency with 1 Counter"=10105, "High Frequency with 2 Counters"=10157, "Large Range with 2 Counters"=10205] ("measurement method")
                  w374 = 10123 items=["Finite Samples"=10178, "Continuous Samples"=10123, "Hardware Timed Single Point"=12522] ("sample mode")
                  # "ctr3"
                  # "ctr2"
                  n166 = call <vilib>:"DAQmx Clear Task.vi"("task in"=w360, "error in"=w361) -> ("error out"=w375:errorcluster)  [unwired: 13 in]
                  n167 = local read "counter 3"() -> (w357:tag)
                  n168 = call <vilib>:"Simple Error Handler.vi"("error in (no error)"=w375) -> ("error out"=w362:errorcluster)  [unwired: 4 in, 4 out]
                  n169 = flat-sequence {
                    tunnel: w359 -> [w376]
                    tunnel: [w376] -> w358
                    frame #0 {
                      n170 = Wait (ms)(milliseconds to wait=u32 2000) -> ()  [unwired: 1 out]
                    }
                  }
                  n171 = local read "counter"() -> (w364:tag)
                  n172 = call <vilib>:"Clear Errors.vi"("error in (no error)"=w362) -> ("error out"=w359:errorcluster)  [unwired: 5 in, 1 out]
                  n173 = Select(t=w364, s=w365, f=w357) -> (s? t:f=w363:tag)
                  n174 = call-poly <vilib>:"DAQmx Create Virtual Channel.vi"("measurement method"=w370, "counter"=w363, "units"=w369, "error in"=w358) -> ("task out"=w372:refnum<k21>, "error out"=w373:errorcluster)  [unwired: 10 in]
                  n175 = call-poly <vilib>:"DAQmx Timing.vi"("task/channels in"=w372, "sample mode"=w374, "error in"=w373) -> ("task out"=w368:refnum<k21>, "error out"=w371:errorcluster)  [unwired: 11 in]
                  n176 = call <vilib>:"DAQmx Start Task.vi"("task/channels in"=w368, "error in"=w371) -> ("task out"=w367:refnum<k21>, "error out"=w366:errorcluster)  [unwired: 12 in]
                }
              }
            }
            frame True {
              n177 = Wait (ms)(milliseconds to wait=u32 2) -> ()  [unwired: 1 out]
              n178 = global read "Global RPM simulati.vi" "Rpm simulati"() -> (w378:dbl)
              n179 = property class="Ring (strict)"(reference="Tipo motore") -> ("Value"=w382:u16)  [unwired: 1 in, 2 out]
              n180 = property class="Clust (strict)"(reference="Dati Targa per calcoli") -> ("Value"=w386:T12)  [unwired: 1 in, 2 out]
              n181 = Unbundle By Name(w386) -> ("trifase.C nom (Nm)"=w385:dbl, "Monofase.C nom (Nm)"=w384:dbl, "Dc.C nom (Nm)"=w379:dbl)
              n182 = Build Array(w378, w378) -> ()  [unwired: 1 out]
              n183 = Build Array(w385, w384, w379, w379) -> (w383:dbl[])
              n184 = Index Array(array=w383, index=w382) -> (element=→"Cnom":dbl)
            }
          }
          "rpm" <- w308
          "error CTR" <- w315
          n185 = case shown="True" w317 {
            tunnel: w319 -> [_ w398]
            tunnel: w308 -> [w390 w392]
            tunnel: w307 -> [w391 w397]
            tunnel: [w389 _] -> w306
            frame False {
              n186 = Build Array (concatenate)(w391, w390) -> (w389:dbl[])
            }
            frame True {
              n187 = call-poly <vilib>:"Mean.vi"("X"=w397) -> ("mean"=w394:dbl)  [unwired: 1 out]
              n188 = Array Size(array=w397) -> (size(s)=w396:i32)
              n189 = Greater Than 0?(x=w396) -> (x > 0?=w395:bool)
              n190 = Select(t=w394, s=w395, f=w392) -> (s? t:f=w393:dbl)
              n191 = Bundle By Name(cluster=cluster{"Stato":string, "dato":variant} {"Stato"="Leggi RPM", "dato"=variant} ("Cluster"), "dato"=w393) -> (w400:cluster{"Stato":string, "dato":variant})
              n192 = Enqueue Element(queue=w398, element=w400) -> ()  [unwired: 2 in, 3 out]
            }
          }
          n193 = global read "EXIT.vi" "EXIT"() -> (w305:bool)
          n194 = Or(x=w315, y=w305) -> (x .or. y?=w314:bool)
        }
        n195 = while {
          shift-right: [w632] -> w221
          shift-left: w222 -> [w634]
          shift-right: [w631] -> w191
          shift-left: w196 -> [w633]
          tunnel: w173 -> [w628]
          tunnel: w172 -> [w625]
          stop <- w630 stop-if-true
          w621 = 26 ("index")
          n196 = case shown="True" w625 {
            tunnel: w634 -> [w772 _]
            tunnel: w633 -> [w771 _]
            tunnel: [w770 _] -> w632
            tunnel: [w769 _] -> w631
            tunnel: [w768 w775] -> w624
            frame False {
              n197 = call-poly <vilib>:"DAQmx Read.vi"("task/channels in"=w772, "error in"=w771) -> ("task out"=w770:refnum<k21>, "data"=w768:bool[], "error out"=w769:errorcluster)  [unwired: 11 in]
            }
            frame True {
              n198 = local read "statoDO"() -> (w774:T11)
              n199 = call "Simula DI.vi"("statoDO_cDaq"=w774) -> ("Stato DI_Cdaq"=w773:T14)  [unwired: 10 in]
              n200 = Cluster To Array(cluster=w773) -> (array=w775:bool[])
            }
          }
          "error DI" <- w631
          n201 = for {
            tunnel: w624 -> [w636] mode=indexing
            tunnel: [w637] -> w622 mode=indexing
            i -> [w639]
            # "filtro per disturbi"
            n202 = Not(x=w636) -> (.not. x?=w635:bool)
            n203 = case shown="16" w639 {
              tunnel: w635 -> [w643 w644 w648 w652 w656 w660 w664 w668 w672 w676 w680 w684 w688 w692 w696 w700 w704 w708 w712 w716 w720 w724 w728 w732 w736 w740 w744 w748 w752 w756 w760 w764]
              tunnel: "Time filtro(s)" -> [w641 w646 w650 w654 w658 w662 w666 w670 w674 w678 w682 w686 w690 w694 w698 w702 w706 w710 w714 w718 w722 w726 w730 w734 w738 w742 w746 w750 w754 w758 w762 w766]
              tunnel: [w640 w645 w649 w653 w657 w661 w665 w669 w673 w677 w681 w685 w689 w693 w697 w701 w705 w709 w713 w717 w721 w725 w729 w733 w737 w741 w745 w749 w753 w757 w761 w765] -> w637
              frame 0, Default {
                n204 = call "Elapsed Time2"("Time Target (s)"=w641, "Reset"=w643, "Auto Reset"=FALSE) -> ("Time has Elapsed"=w640:bool)  [unwired: 9 in, 7 out]
              }
              frame 1 {
                n205 = call "Elapsed Time3"("Time Target (s)"=w646, "Reset"=w644, "Auto Reset"=FALSE) -> ("Time has Elapsed"=w645:bool)  [unwired: 9 in, 7 out]
              }
              frame 2 {
                n206 = call "Elapsed Time4"("Time Target (s)"=w650, "Reset"=w648, "Auto Reset"=FALSE) -> ("Time has Elapsed"=w649:bool)  [unwired: 9 in, 7 out]
              }
              frame 3 {
                n207 = call "Elapsed Time5"("Time Target (s)"=w654, "Reset"=w652, "Auto Reset"=FALSE) -> ("Time has Elapsed"=w653:bool)  [unwired: 9 in, 7 out]
              }
              frame 4 {
                n208 = call "Elapsed Time6"("Time Target (s)"=w658, "Reset"=w656, "Auto Reset"=FALSE) -> ("Time has Elapsed"=w657:bool)  [unwired: 9 in, 7 out]
              }
              frame 5 {
                n209 = call "Elapsed Time7"("Time Target (s)"=w662, "Reset"=w660, "Auto Reset"=FALSE) -> ("Time has Elapsed"=w661:bool)  [unwired: 9 in, 7 out]
              }
              frame 6 {
                n210 = call "Elapsed Time8"("Time Target (s)"=w666, "Reset"=w664, "Auto Reset"=FALSE) -> ("Time has Elapsed"=w665:bool)  [unwired: 9 in, 7 out]
              }
              frame 7 {
                n211 = call "Elapsed Time9"("Time Target (s)"=w670, "Reset"=w668, "Auto Reset"=FALSE) -> ("Time has Elapsed"=w669:bool)  [unwired: 9 in, 7 out]
              }
              frame 8 {
                n212 = call "Elapsed Time10"("Time Target (s)"=w674, "Reset"=w672, "Auto Reset"=FALSE) -> ("Time has Elapsed"=w673:bool)  [unwired: 9 in, 7 out]
              }
              frame 9 {
                n213 = call "Elapsed Time11"("Time Target (s)"=w678, "Reset"=w676, "Auto Reset"=FALSE) -> ("Time has Elapsed"=w677:bool)  [unwired: 9 in, 7 out]
              }
              frame 10 {
                n214 = call "Elapsed Time12"("Time Target (s)"=w682, "Reset"=w680, "Auto Reset"=FALSE) -> ("Time has Elapsed"=w681:bool)  [unwired: 9 in, 7 out]
              }
              frame 11 {
                n215 = call "Elapsed Time13"("Time Target (s)"=w686, "Reset"=w684, "Auto Reset"=FALSE) -> ("Time has Elapsed"=w685:bool)  [unwired: 9 in, 7 out]
              }
              frame 12 {
                n216 = call "Elapsed Time14"("Time Target (s)"=w690, "Reset"=w688, "Auto Reset"=FALSE) -> ("Time has Elapsed"=w689:bool)  [unwired: 9 in, 7 out]
              }
              frame 13 {
                n217 = call "Elapsed Time15"("Time Target (s)"=w694, "Reset"=w692, "Auto Reset"=FALSE) -> ("Time has Elapsed"=w693:bool)  [unwired: 9 in, 7 out]
              }
              frame 14 {
                n218 = call "Elapsed Time16"("Time Target (s)"=w698, "Reset"=w696, "Auto Reset"=FALSE) -> ("Time has Elapsed"=w697:bool)  [unwired: 9 in, 7 out]
              }
              frame 15 {
                n219 = call "Elapsed Time17"("Time Target (s)"=w702, "Reset"=w700, "Auto Reset"=FALSE) -> ("Time has Elapsed"=w701:bool)  [unwired: 9 in, 7 out]
              }
              frame 16 {
                n220 = call "Elapsed Time18"("Time Target (s)"=w706, "Reset"=w704, "Auto Reset"=FALSE) -> ("Time has Elapsed"=w705:bool)  [unwired: 9 in, 7 out]
              }
              frame 17 {
                n221 = call "Elapsed Time19"("Time Target (s)"=w710, "Reset"=w708, "Auto Reset"=FALSE) -> ("Time has Elapsed"=w709:bool)  [unwired: 9 in, 7 out]
              }
              frame 18 {
                n222 = call "Elapsed Time20"("Time Target (s)"=w714, "Reset"=w712, "Auto Reset"=FALSE) -> ("Time has Elapsed"=w713:bool)  [unwired: 9 in, 7 out]
              }
              frame 19 {
                n223 = call "Elapsed Time21"("Time Target (s)"=w718, "Reset"=w716, "Auto Reset"=FALSE) -> ("Time has Elapsed"=w717:bool)  [unwired: 9 in, 7 out]
              }
              frame 20 {
                n224 = call "Elapsed Time22"("Time Target (s)"=w722, "Reset"=w720, "Auto Reset"=FALSE) -> ("Time has Elapsed"=w721:bool)  [unwired: 9 in, 7 out]
              }
              frame 21 {
                n225 = call "Elapsed Time23"("Time Target (s)"=w726, "Reset"=w724, "Auto Reset"=FALSE) -> ("Time has Elapsed"=w725:bool)  [unwired: 9 in, 7 out]
              }
              frame 22 {
                n226 = call "Elapsed Time24"("Time Target (s)"=w730, "Reset"=w728, "Auto Reset"=FALSE) -> ("Time has Elapsed"=w729:bool)  [unwired: 9 in, 7 out]
              }
              frame 23 {
                n227 = call "Elapsed Time25"("Time Target (s)"=w734, "Reset"=w732, "Auto Reset"=FALSE) -> ("Time has Elapsed"=w733:bool)  [unwired: 9 in, 7 out]
              }
              frame 24 {
                n228 = call "Elapsed Time26"("Time Target (s)"=w738, "Reset"=w736, "Auto Reset"=FALSE) -> ("Time has Elapsed"=w737:bool)  [unwired: 9 in, 7 out]
              }
              frame 25 {
                n229 = call "Elapsed Time27"("Time Target (s)"=w742, "Reset"=w740, "Auto Reset"=FALSE) -> ("Time has Elapsed"=w741:bool)  [unwired: 9 in, 7 out]
              }
              frame 26 {
                n230 = call "Elapsed Time28"("Time Target (s)"=w746, "Reset"=w744, "Auto Reset"=FALSE) -> ("Time has Elapsed"=w745:bool)  [unwired: 9 in, 7 out]
              }
              frame 27 {
                n231 = call "Elapsed Time29"("Time Target (s)"=w750, "Reset"=w748, "Auto Reset"=FALSE) -> ("Time has Elapsed"=w749:bool)  [unwired: 9 in, 7 out]
              }
              frame 28 {
                n232 = call "Elapsed Time30"("Time Target (s)"=w754, "Reset"=w752, "Auto Reset"=FALSE) -> ("Time has Elapsed"=w753:bool)  [unwired: 9 in, 7 out]
              }
              frame 29 {
                n233 = call "Elapsed Time31"("Time Target (s)"=w758, "Reset"=w756, "Auto Reset"=FALSE) -> ("Time has Elapsed"=w757:bool)  [unwired: 9 in, 7 out]
              }
              frame 30 {
                n234 = call "Elapsed Time32"("Time Target (s)"=w762, "Reset"=w760, "Auto Reset"=FALSE) -> ("Time has Elapsed"=w761:bool)  [unwired: 9 in, 7 out]
              }
              frame 31 {
                n235 = call "Elapsed Time33"("Time Target (s)"=w766, "Reset"=w764, "Auto Reset"=FALSE) -> ("Time has Elapsed"=w765:bool)  [unwired: 9 in, 7 out]
              }
            }
          }
          n236 = Index Array(array=w622, index=w621) -> (element=w623:bool)
          n237 = Not(x=w623) -> (.not. x?=w620:bool)
          n238 = Replace Array Subset(array=w622, new element=w620, index=w621) -> (w619:bool[])
          n239 = Array To Cluster(array=w619) -> ()  [unwired: 1 out]
          n240 = Bundle By Name(cluster=cluster{"Stato":string, "dato":variant} {"Stato"="Leggi DI cDAQ", "dato"=variant} ("Cluster"), "dato"=w619) -> (w626:cluster{"Stato":string, "dato":variant})
          n241 = global read "EXIT.vi" "EXIT"() -> (w618:bool)
          n242 = Enqueue Element(queue=w628, element=w626) -> ()  [unwired: 2 in, 3 out]
          n243 = Or(x=w631, y=w618) -> (x .or. y?=w630:bool)
          n244 = Wait Until Next ms Multiple(millisecond multiple=u32 100) -> ()  [unwired: 1 out]
        }
        n245 = while {
          shift-right: [w604] -> w220
          shift-left: w216 -> [w606]
          shift-right: [w603] -> w219
          shift-left: w197 -> [w605]
          tunnel: w173 -> [w599]
          tunnel: w172 -> [w596]
          stop <- w595 stop-if-true
          n246 = case shown="True" w596 {
            tunnel: w606 -> [w611 _]
            tunnel: w605 -> [w610 _]
            tunnel: [w609 _] -> w604
            tunnel: [w608 _] -> w603
            tunnel: [w607 w612] -> w598
            frame False {
              n247 = call-poly <vilib>:"DAQmx Read.vi"("task/channels in"=w611, "error in"=w610) -> ("task out"=w609:refnum<k21>, "data"=w607:dbl[], "error out"=w608:errorcluster)  [unwired: 11 in]
            }
            frame True {
              n248 = for {
                N: 8 -> [_]
                tunnel: 25.0 -> [w617]
                tunnel: [w615] -> w612 mode=indexing
                n249 = Random Number (0-1)() -> (number: 0 to 1=w616:dbl)
                n250 = Add(x=w617, y=w616) -> (x+y=w615:dbl)
              }
            }
          }
          "error TC" <- w603
          n251 = Array To Cluster(array=w598) -> (cluster=→"Termocoppie":T15)
          n252 = Bundle By Name(cluster=cluster{"Stato":string, "dato":variant} {"Stato"="Leggi TC", "dato"=variant} ("Cluster"), "dato"=w598) -> (w600:cluster{"Stato":string, "dato":variant})
          n253 = global read "EXIT.vi" "EXIT"() -> (w594:bool)
          n254 = Enqueue Element(queue=w599, element=w600) -> ()  [unwired: 2 in, 3 out]
          n255 = Or(x=w603, y=w594) -> (x .or. y?=w595:bool)
          n256 = Wait Until Next ms Multiple(millisecond multiple=u32 100) -> ()  [unwired: 1 out]
        }
        n257 = while {
          shift-right: [w531] -> w209
          shift-left: w208 -> [w532]
          shift-right: [w521] -> w192
          shift-left: w195 -> [w530]
          tunnel: w173 -> [w527]
          tunnel: w205 -> [w525]
          tunnel: w206 -> [w524]
          tunnel: w172 -> [w519]
          shift-right: [w516] -> _
          shift-left: w182 -> [w515]
          shift-right: [w511] -> _
          shift-left: _ -> [w512]
          stop <- w510 stop-if-true
          n258 = Dequeue Element(queue=w525, error in (no error)=w524) -> (queue out=w523:refnum<queue>, element=w526:dbl[])  [unwired: 1 in, 2 out]
          n259 = for {
            tunnel: w526 -> [w562] mode=indexing
            tunnel: [w561] -> w514 mode=indexing
            n260 = In Range and Coerce(upper limit=10.0, x=w562, lower limit=0.0) -> (coerced(x)=w561:dbl)  [unwired: 1 out]
          }
          n261 = Get Queue Status(queue=w523) -> (# elements in queue=→"# pending insert 2":i32)  [unwired: 2 in, 7 out]
          n262 = Equal?(x=w514, y=w515) -> (x = y?=w517:bool)
          n263 = Array To Cluster(array=w515) -> (cluster=→"statoAO":T13)
          n264 = Bundle By Name(cluster=cluster{"Stato":string, "dato":variant} {"Stato"="Stato AO cDAQ", "dato"=variant} ("Cluster"), "dato"=w514) -> (w528:cluster{"Stato":string, "dato":variant})
          n265 = Enqueue Element(queue=w527, element=w528) -> ()  [unwired: 2 in, 3 out]
          n266 = Tick Count (ms)() -> (millisecond timer value=w511:u32)
          n267 = Subtract(x=w511, y=w512) -> (x-y=→"t ciclo effettivo AO":u32)
          n268 = global read "EXIT.vi" "EXIT"() -> (w509:bool)
          n269 = Compound Arithmetic op=OR(w517, w519, w509) -> (w518:bool)
          n270 = case shown="False" w518 {
            tunnel: w532 -> [w545 w559]
            tunnel: [w544 w559] -> w531
            tunnel: w530 -> [w543 w558]
            tunnel: [w542 w558] -> w521
            tunnel: w514 -> [w541 w560]
            tunnel: [w541 w560] -> w516
            frame False {
              n271 = flat-sequence {
                tunnel: w541 -> [w547]
                tunnel: w543 -> [w548]
                tunnel: w545 -> [w549]
                tunnel: [w549] -> w540
                tunnel: [w548] -> w539
                tunnel: [w547] -> w538
                tunnel: [w546] -> w534
                tunnel: w540 -> [w554]
                tunnel: w539 -> [w552]
                tunnel: w538 -> [w550]
                tunnel: [w553] -> w537
                tunnel: [w551] -> w536
                tunnel: [w556] -> w542
                tunnel: [w557] -> w544
                tunnel: w537 -> [w557]
                tunnel: w536 -> [w556]
                tunnel: [w555] -> w535
                frame #0 {
                  n272 = Tick Count (ms)() -> (millisecond timer value=w546:u32)
                }
                frame #1 {
                  n273 = call-poly <vilib>:"DAQmx Write.vi"("task/channels in"=w554, "data"=w550, "error in"=w552) -> ("task out"=w553:refnum<k21>, "error out"=w551:errorcluster)  [unwired: 10 in, 1 out]
                }
                frame #2 {
                  n274 = Tick Count (ms)() -> (millisecond timer value=w555:u32)
                }
              }
              n275 = Subtract(x=w535, y=w534) -> (x-y=→"x-y":u32)
            }
            frame True {
            }
          }
          "error AO" <- w521
          n276 = Or(x=w521, y=w509) -> (x .or. y?=w510:bool)
        }
        n277 = while {
          shift-right: [w584] -> w217
          shift-left: w218 -> [w585]
          shift-right: [w567] -> w193
          shift-left: w194 -> [w583]
          tunnel: w173 -> [w580]
          tunnel: w210 -> [w578]
          tunnel: w211 -> [w579]
          tunnel: w172 -> [w572]
          shift-right: [w569] -> _
          shift-left: bool[] [] -> [w568]
          i -> [w576]
          stop <- w566 stop-if-true
          n278 = Dequeue Element(queue=w578, error in (no error)=w579) -> (queue out=w577:refnum<queue>, element=w573:bool[])  [unwired: 1 in, 2 out]
          n279 = global read "EXIT.vi" "EXIT"() -> (w565:bool)
          n280 = Get Queue Status(queue=w577) -> (# elements in queue=→"# pending insert":i32)  [unwired: 2 in, 7 out]
          n281 = Equal?(x=w568, y=w573) -> (x = y?=w571:bool)
          n282 = Array To Cluster(array=w568) -> (cluster=→"statoDO":T16)
          n283 = Compound Arithmetic op=OR(w571, w572, w565) -> (w570:bool)
          n284 = Bundle By Name(cluster=cluster{"Stato":string, "dato":variant} {"Stato"="Stato DO cDAQ", "dato"=variant} ("Cluster"), "dato"=w573) -> (w581:cluster{"Stato":string, "dato":variant})
          n285 = case shown="False" w570 {
            tunnel: w585 -> [w590 w592]
            tunnel: [w589 w592] -> w584
            tunnel: w583 -> [w588 w591]
            tunnel: [w587 w591] -> w567
            tunnel: w573 -> [w586 w593]
            tunnel: [w586 w593] -> w569
            frame False {
              n286 = call-poly <vilib>:"DAQmx Write.vi"("task/channels in"=w590, "data"=w586, "error in"=w588) -> ("task out"=w589:refnum<k21>, "error out"=w587:errorcluster)  [unwired: 10 in, 1 out]
            }
            frame True {
            }
          }
          "error DO" <- w567
          n287 = Enqueue Element(queue=w580, element=w581) -> ()  [unwired: 2 in, 3 out]
          n288 = Or(x=w567, y=w565) -> (x .or. y?=w566:bool)
          "Numeric" <- w576
        }
        n289 = call <vilib>:"DAQmx Clear Task.vi"("task in"=w217, "error in"=w193) -> ("error out"=w186:errorcluster)  [unwired: 13 in]
        n290 = call <vilib>:"Simple Error Handler.vi"("error in (no error)"=w186) -> ()  [unwired: 4 in, 5 out]
        n291 = call <vilib>:"DAQmx Clear Task.vi"("task in"=w179, "error in"=w180) -> ("error out"=w181:errorcluster)  [unwired: 13 in]
        n292 = call <vilib>:"DAQmx Clear Task.vi"("task in"=w177, "error in"=w178) -> ("error out"=w176:errorcluster)  [unwired: 13 in]
        n293 = call <vilib>:"DAQmx Clear Task.vi"("task in"=w209, "error in"=w192) -> ("error out"=w187:errorcluster)  [unwired: 13 in]
        n294 = call <vilib>:"DAQmx Clear Task.vi"("task in"=w221, "error in"=w191) -> ("error out"=w188:errorcluster)  [unwired: 13 in]
        n295 = call <vilib>:"DAQmx Clear Task.vi"("task in"=w220, "error in"=w219) -> ("error out"=w189:errorcluster)  [unwired: 13 in]
        n296 = call <vilib>:"DAQmx Clear Task.vi"("task in"=w214, "error in"=w215) -> ("error out"=w190:errorcluster)  [unwired: 13 in]
        n297 = call <vilib>:"Simple Error Handler.vi"("error in (no error)"=w181) -> ()  [unwired: 4 in, 5 out]
        n298 = call <vilib>:"Simple Error Handler.vi"("error in (no error)"=w187) -> ()  [unwired: 4 in, 5 out]
        n299 = call <vilib>:"Simple Error Handler.vi"("error in (no error)"=w176) -> ()  [unwired: 4 in, 5 out]
        n300 = call <vilib>:"Simple Error Handler.vi"("error in (no error)"=w189) -> ()  [unwired: 4 in, 5 out]
        n301 = call <vilib>:"Simple Error Handler.vi"("error in (no error)"=w188) -> ()  [unwired: 4 in, 5 out]
        n302 = call <vilib>:"Simple Error Handler.vi"("error in (no error)"=w190) -> ()  [unwired: 4 in, 5 out]
      }
      frame "EXIT" {
        n303 = Release Queue(queue=w778) -> ()  [unwired: 2 in, 3 out]
        n304 = property on="EXIT" class="Bool (strict)"("Val(Sgnl)"=TRUE ("Value (Signaling)")) -> ()  [unwired: 2 in, 2 out]
      }
    }
    "String" <- w34
  }
  "error out" <- w3
  n305 = local write "stop"(FALSE ("stop")) -> ()
  n306 = global write "EXIT.vi" "EXIT"(FALSE ("EXIT")) -> ()
  n307 = while {
    stop <- w779 stop-if-true
    n308 = event shown="[3] \"EXIT\": Value Change" {
      selector: _ -> [_ _ _ _]
      dyn-events: _ -> [_ _ _ _]
      timeout: _ -> [_ _ _ _]
      tunnel: [_ _ _ TRUE] -> w779
      event Timeout {
        n309 = event-data() -> ()  [unwired: 1 in, 3 out]
      }
      event "SET DO": Value Change {
        n310 = event-data() -> ()  [unwired: 1 in, 4 out]
        n311 = call "Set DO.vi"("Cluster SET DO"="Array DO") -> ()  [unwired: 10 in, 1 out]
      }
      event "SET AO": Value Change {
        n312 = event-data() -> ()  [unwired: 1 in, 4 out]
        n313 = call "SET AO.vi"("Cluster SET AO"="Cluster SET AO") -> ()  [unwired: 10 in, 1 out]
      }
      event "EXIT": Value Change {
        n314 = event-data() -> ()  [unwired: 1 in, 4 out]
        n315 = Bundle By Name(cluster=T3 {"AO"=enum."OFF: ALL AO", "Value"=0.0} ("Cluster SET AO"), "AO"=9999) -> (w785:T3)
        n316 = Build Array(w785) -> (w788:T3[])
        n317 = call "Set DO.vi"("Cluster SET DO"=T5 [{"DO"=enum."Exit", "Value"=FALSE}]) -> ()  [unwired: 10 in, 1 out]
        n318 = call "SET AO.vi"("Cluster SET AO"=w788) -> ()  [unwired: 10 in, 1 out]
        n319 = global write "EXIT.vi" "EXIT"(TRUE ("EXIT")) -> ()
        n320 = local write "stop"(TRUE ("stop")) -> ()
      }
    }
  }
